vi "Multi U-Link DAQ Continuous value.vi"() -> ()   [LabVIEW 2017]
doc: "by Tanguy BOULARD"
uses:
  Type Def/Data.ctl
  <vilib>/Analysis/NI_AALBase.lvlib
panel:
  out "Energie IR file (500pts)":refnum<file>
  out "Puissance depolar file (500pts)":refnum<file>
  out "Energy UV file (500pts)":refnum<file>
  out "stop IR":bool
  out "stop Pd":bool
  out "stop UV":bool
  out "12sec IR":bool
  out "12sec Pd":bool
  out "12sec UV":bool
  out "Tableau IR":dbl[](array[numeric])
  out "Tableau UV":dbl[](array[numeric])
  out "Tableau Puissance depolar":dbl[](array[numeric])
  out "taille IR":dbl format="%.2f"
  out "taille Pd":dbl format="%.2f"
  out "taille UV":dbl format="%.2f"
  out "Energie IR mean":dbl caption="moyenne" format="%g"
  out "Energie IR variance":dbl caption="variance" format="%g"
  out "Energie IR max":dbl caption="max" format="%#_5g"
  out "Energie IR min":dbl caption="min"
  out "Puissance depolar mean":dbl caption="moyenne" format="%g"
  out "Puissance depolar variance":dbl caption="variance" format="%g"
  out "Puissance depolar max":dbl caption="max" format="%#_5g"
  out "Puissance depolar min":dbl caption="min" format="%#_5g"
  out "Energie UV mean":dbl caption="moyenne" format="%g"
  out "Energie UV variance":dbl caption="variance" format="%g"
  out "Energie UV max":dbl caption="max" format="%#_5g"
  out "Energie UV min":dbl caption="min" format="%#_5g"
  out "Energie UV rapport":dbl caption="rapport" format="%#_5g"
  out "Puissance depolar rapport":dbl caption="rapport" format="%#_5g"
  out "Energie IR rapport":dbl caption="rapport" format="%#_5g"
  out "Chaîne":string="Energie UV"
  out "Chaîne 2":string="Puissance depolar"
  out "Chaîne 3":string="Energie IR"
  out "sortie d'erreur":errorcluster caption="Sortie d'erreur"
  in  "stop":bool
  out "Energie IR value":dbl format="%#_4f"
  out "Energie IR graph":dbl(graph)
  out "Puissance depolar value":dbl format="%#_4f"
  out "Puissance depolar graph":dbl(graph)
  out "Energie IR table":dbl[](array[numeric])
  out "Energie IR table (1sec)":dbl[](array[numeric])
  out "Puissance depolar table":dbl[](array[numeric])
  out "Energie UV value":dbl format="%#_4f"
  out "Energie UV graph":dbl(graph)
  out "Energie UV table":dbl[](array[numeric])
  out "Energie UV table(1sec)":dbl[](array[numeric])
  out "Taux depolar value":dbl format="%#_4f"
  out "taux depolar graph":dbl(graph)
  out "Puissance depolar table (stats)":dbl[][](array[numeric])
  out "Energie IR table (stats)":dbl[][](array[numeric])
  out "Taux depolar indicator":u32(colorbox)=16777222
  out "Puissance depolar table (1sec)":dbl[](array[numeric])
  out "Energie UV table (stats)":dbl[][](array[numeric])
  out "timer 1sec":bool
  out "timer 12sec":bool
  in  "1sec":bool
  in  "12sec":bool
  out "index 1sec":i32
  out "index 12sec":i32
  out "Chaîne 4":string="Energie UV (mJ)"
  out "Chaîne 5":string="Energie IR (mJ)"
  out "Chaîne 6":string="Puissance depolar (W)"
  out "Chaîne 7":string="Taux depolar"
  out "Update":string="Initialization : matching U-Link ports, creating data file"
  in  "Start acquisition":bool
  in  "Commande onglets":T1(tab)
  out "Ressource VISA (Energie UV)":refnum<visa-resource-name>
  out "Wavelength (nm) (Energie UV)":u32=355
  out "Offset (Energie UV)":sgl
  out "Multiplier (Energie UV)":sgl=1.0
  out "Trigger Level (% of Scale) (Energie UV)":dbl=2.0 min=0.1 max=99.9 step=0.1 format="%_3f"
  out "Auto Scale (Energie UV)":bool=TRUE
  out "File name (Energie UV)":string="data.csv"
  out "Scale (Watt or Joule) (Energie UV)":i32(ring) items=["1 pico", "3 pico", "10 pico", "30 pico", "100 pico", "300 pico", "1 nano", "3 nano", "10 nano", "30 nano", "100 nano", "300 nano", "1 micro", "3 micro", "10 micro", "30 micro", "100 micro", "300 micro", "1 milli", "3 milli", "10 milli", "30 milli", "100 milli", "300 milli", "1", "3", "10", "30", "100", "300", "1 kilo", "3 kilo", "10 kilo", "30 kilo", "100 kilo", "300 kilo", "1 mega", "3 mega", "10 mega", "30 mega", "100 mega", "300 mega"]
  out "Ressource VISA (Puissance depolar)":refnum<visa-resource-name>
  out "Offset (Puissance depolar)":sgl
  out "Wavelength (nm) (Puissance depolar)":u32=1064
  out "Multiplier (Puissance depolar)":sgl=1.0
  out "Trigger Level (% of Scale) (Puissance depolar)":dbl=2.0 min=0.1 max=99.9 step=0.1 format="%_3f"
  out "Auto Scale (Puissance depolar)":bool=TRUE
  out "File name (Puissance depolar)":string="data.csv"
  out "Scale (Watt or Joule) (Puissance depolar)":u16(ring) items=["1 pico", "3 pico", "10 pico", "30 pico", "100 pico", "300 pico", "1 nano", "3 nano", "10 nano", "30 nano", "100 nano", "300 nano", "1 micro", "3 micro", "10 micro", "30 micro", "100 micro", "300 micro", "1 milli", "3 milli", "10 milli", "30 milli", "100 milli", "300 milli", "1", "3", "10", "30", "100", "300", "1 kilo", "3 kilo", "10 kilo", "30 kilo", "100 kilo", "300 kilo", "1 mega", "3 mega", "10 mega", "30 mega", "100 mega", "300 mega"]
  out "Ressource VISA (Energie IR)":refnum<visa-resource-name>
  out "Wavelength (nm) (Energie IR)":u32=1064
  out "Offset (Energie IR)":sgl
  out "Multiplier (Energie IR)":sgl=1.0
  out "Trigger Level (% of Scale) (Energie IR)":dbl=2.0 min=0.1 max=99.9 step=0.1 format="%_3f"
  out "File name (Energie IR)":string="data.csv"
  out "Scale (Watt or Joule) (Energie IR)":u16(ring) items=["1 pico", "3 pico", "10 pico", "30 pico", "100 pico", "300 pico", "1 nano", "3 nano", "10 nano", "30 nano", "100 nano", "300 nano", "1 micro", "3 micro", "10 micro", "30 micro", "100 micro", "300 micro", "1 milli", "3 milli", "10 milli", "30 milli", "100 milli", "300 milli", "1", "3", "10", "30", "100", "300", "1 kilo", "3 kilo", "10 kilo", "30 kilo", "100 kilo", "300 kilo", "1 mega", "3 mega", "10 mega", "30 mega", "100 mega", "300 mega"]
  out "Auto Scale (Energie IR)":bool
  out "error IO":errorcluster
  out "COM Port table":refnum<visa-resource-name>[](array[refnum])
  out "COM Port (Energie IR)":i64
  out "COM Port (Puissance depolar)":i64
  out "COM port (Energie UV)":i64
  out "User file contents Energie UV":dbl[](array[numeric])
  out "User file contents Energie IR":dbl[](array[numeric])
  out "User file contents Puissance depolar":dbl[](array[numeric])
  out "error?":bool caption="erreur ?"
  out "file path":path
  out "sortie d'erreur 3":errorcluster caption="sortie d'erreur"
  out "sortie d'erreur 2":errorcluster caption="sortie d'erreur"
  out "Energie UV file (1sec)":refnum<file>
  out "Energie UV file (stats)":refnum<file>
  out "Puissance depolar file (1sec)":refnum<file>
  out "Puissance depolar file (stats)":refnum<file>
  out "Energie IR file (1sec)":refnum<file>
  out "Energie IR file (stats)":refnum<file>
  in  "Bouton Accueil":bool
  out "chaîne de date/heure":string
  out "valeur de l'horloge en ms":u32
  out "Time":string
  out "stop?":bool=TRUE
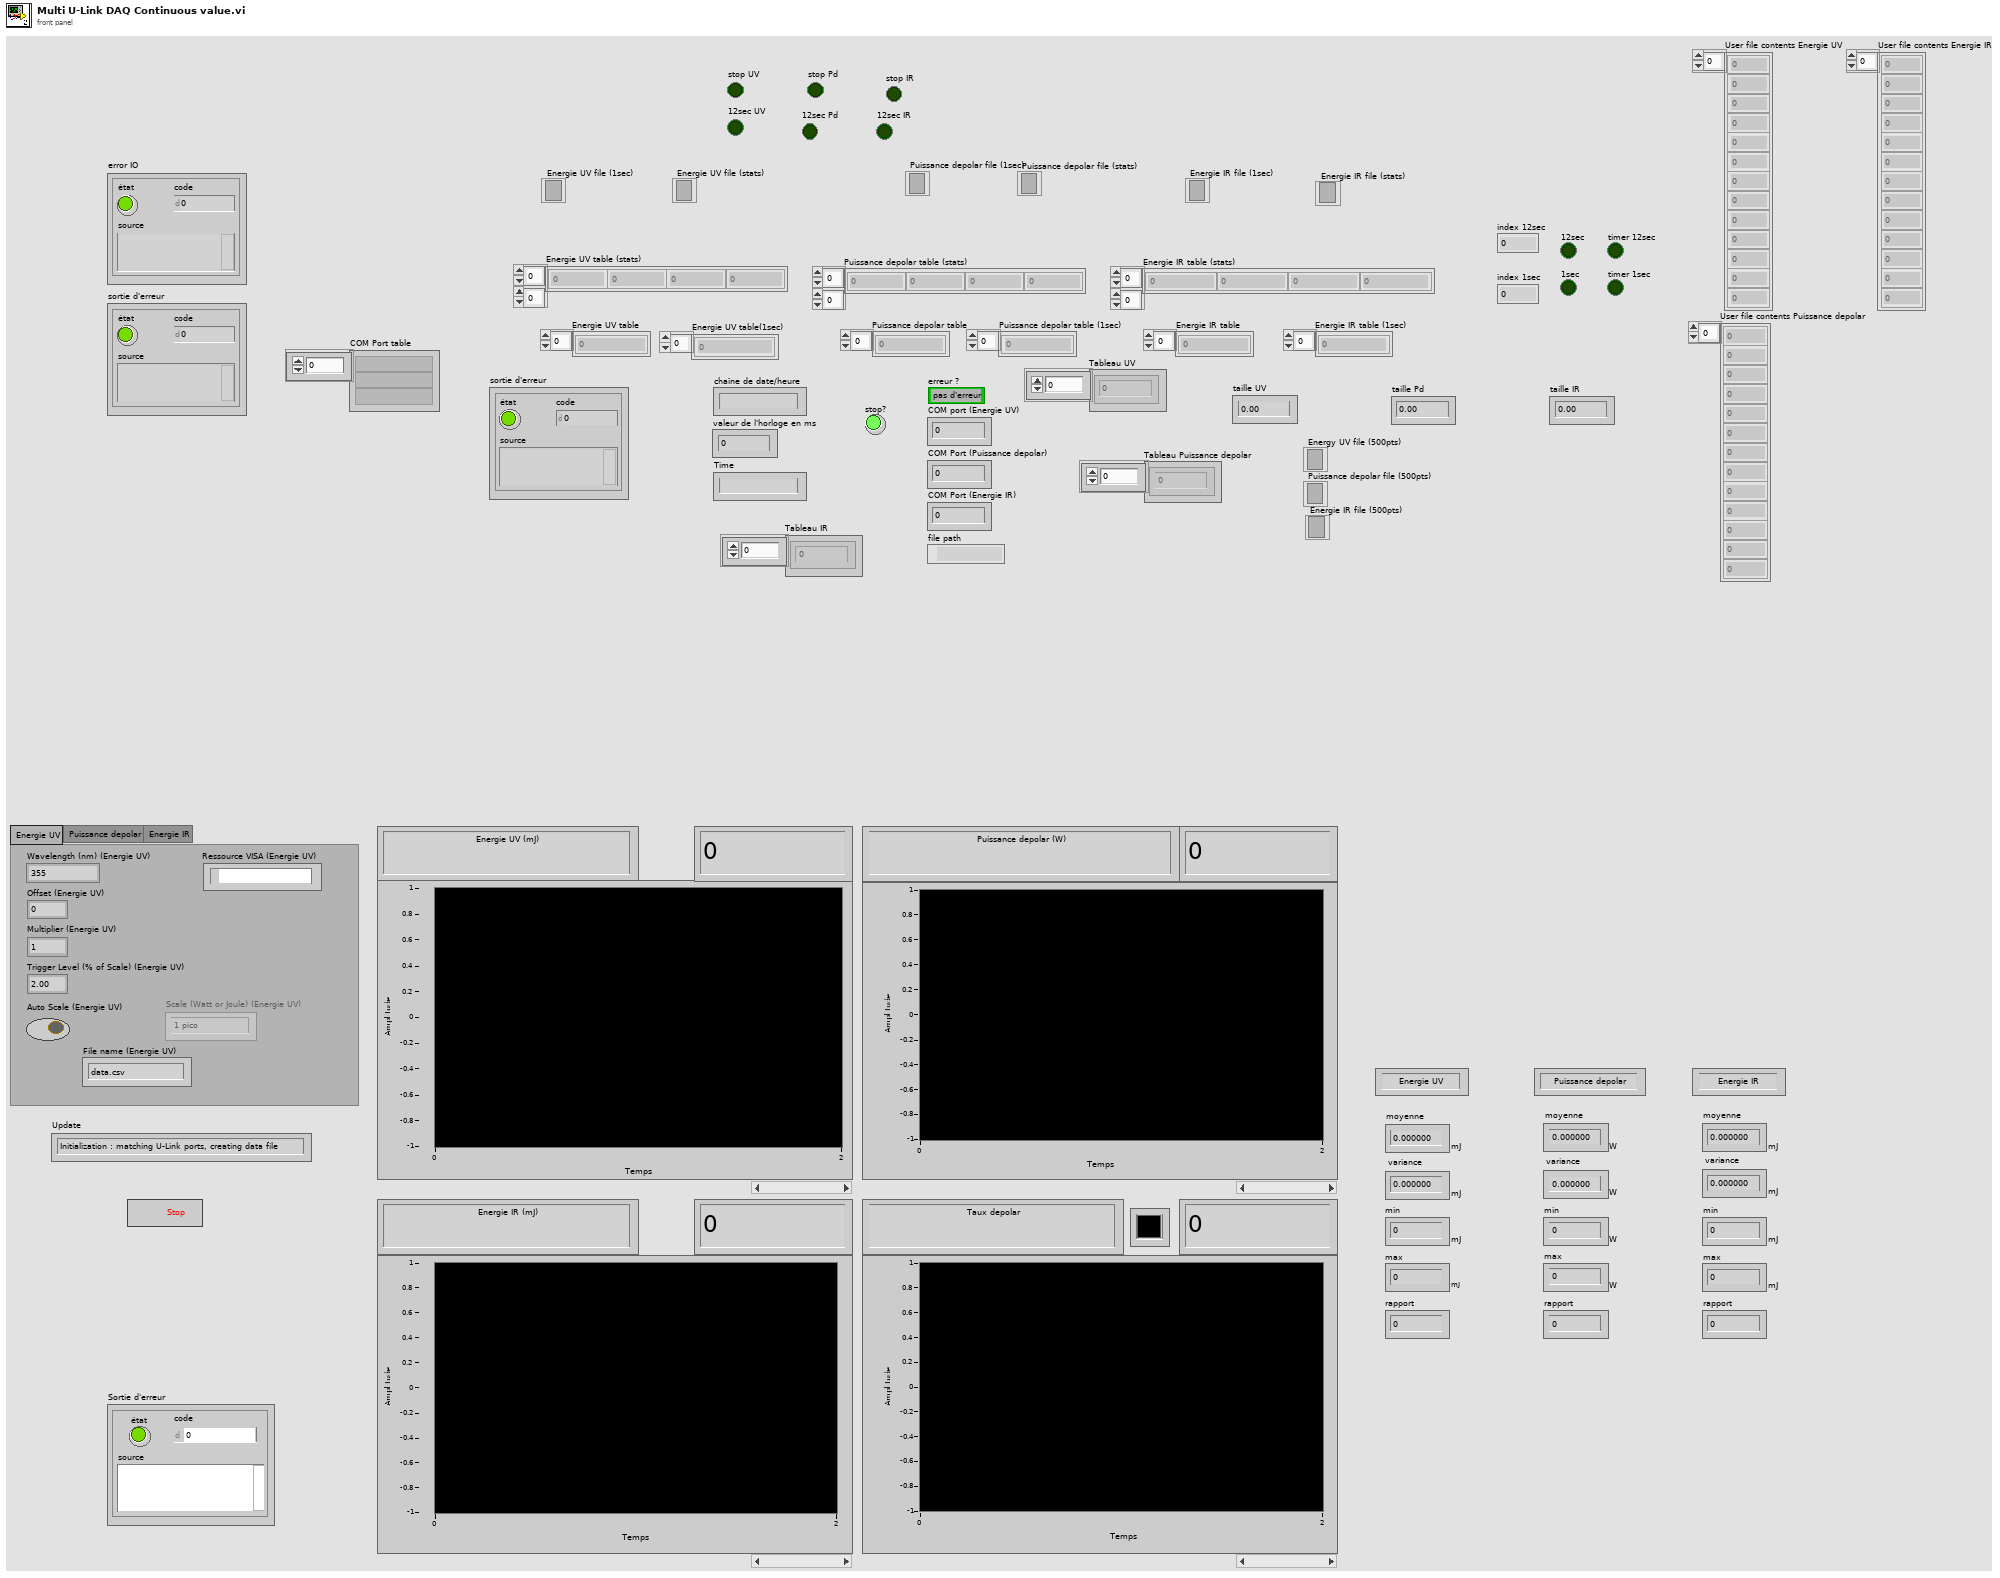
[diagram p1: front panel]
types:
  T1 = enum32{"Energie UV", "Puissance depolar", "Energie IR"}
  T2 = enum8{"Enabled", "Disabled", "Disabled and Grayed Out"}
  T3 = typedef "Data.ctl" = cluster{enum16{"Init", "Read", "Stop", "12sec"}, "Data":dbl}
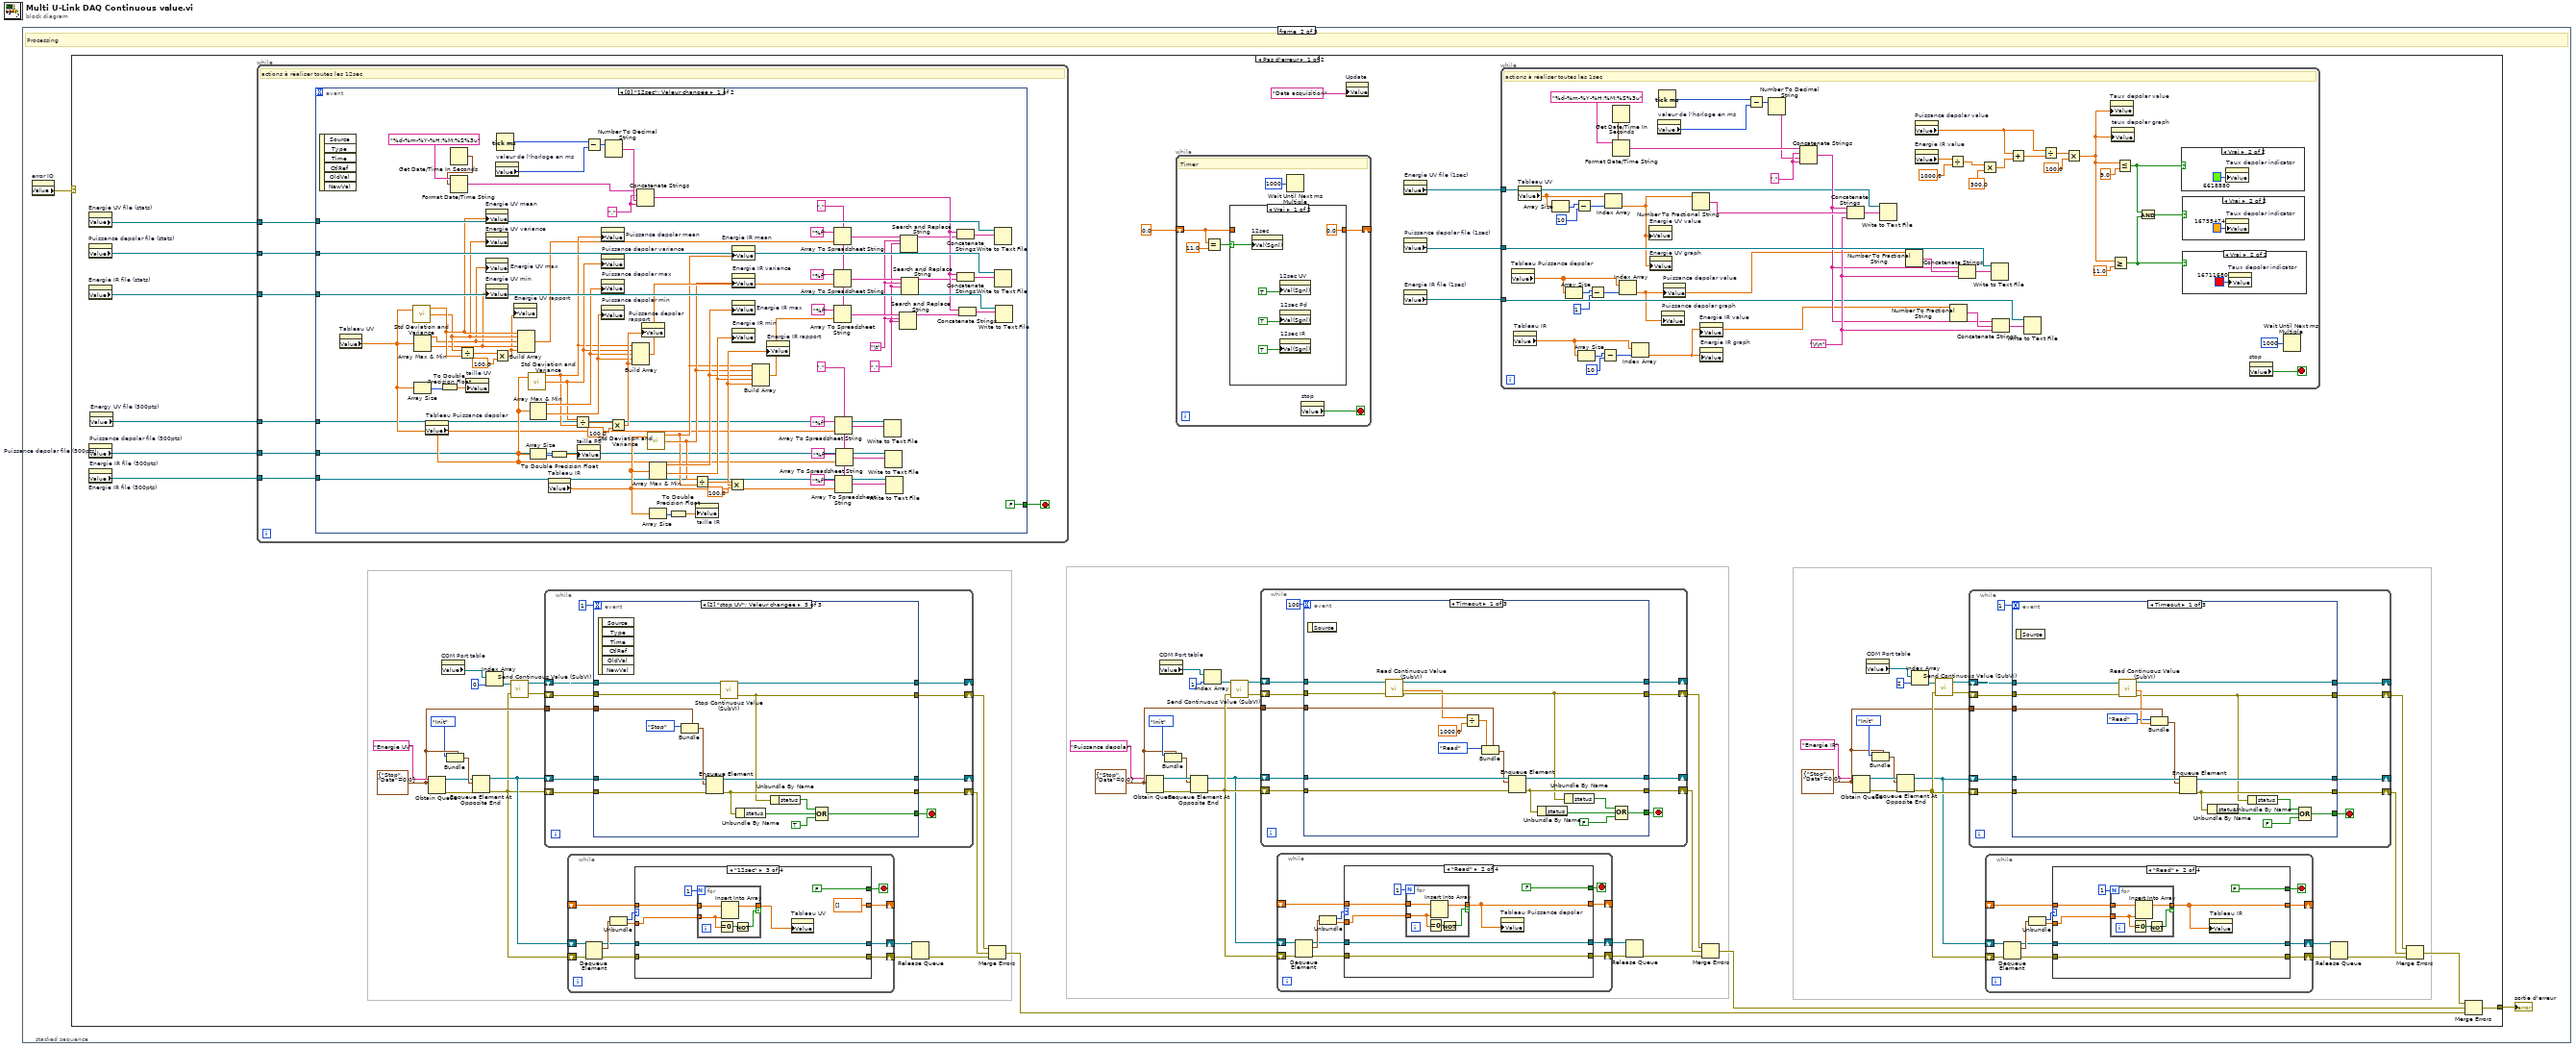
[diagram p0: block diagram]
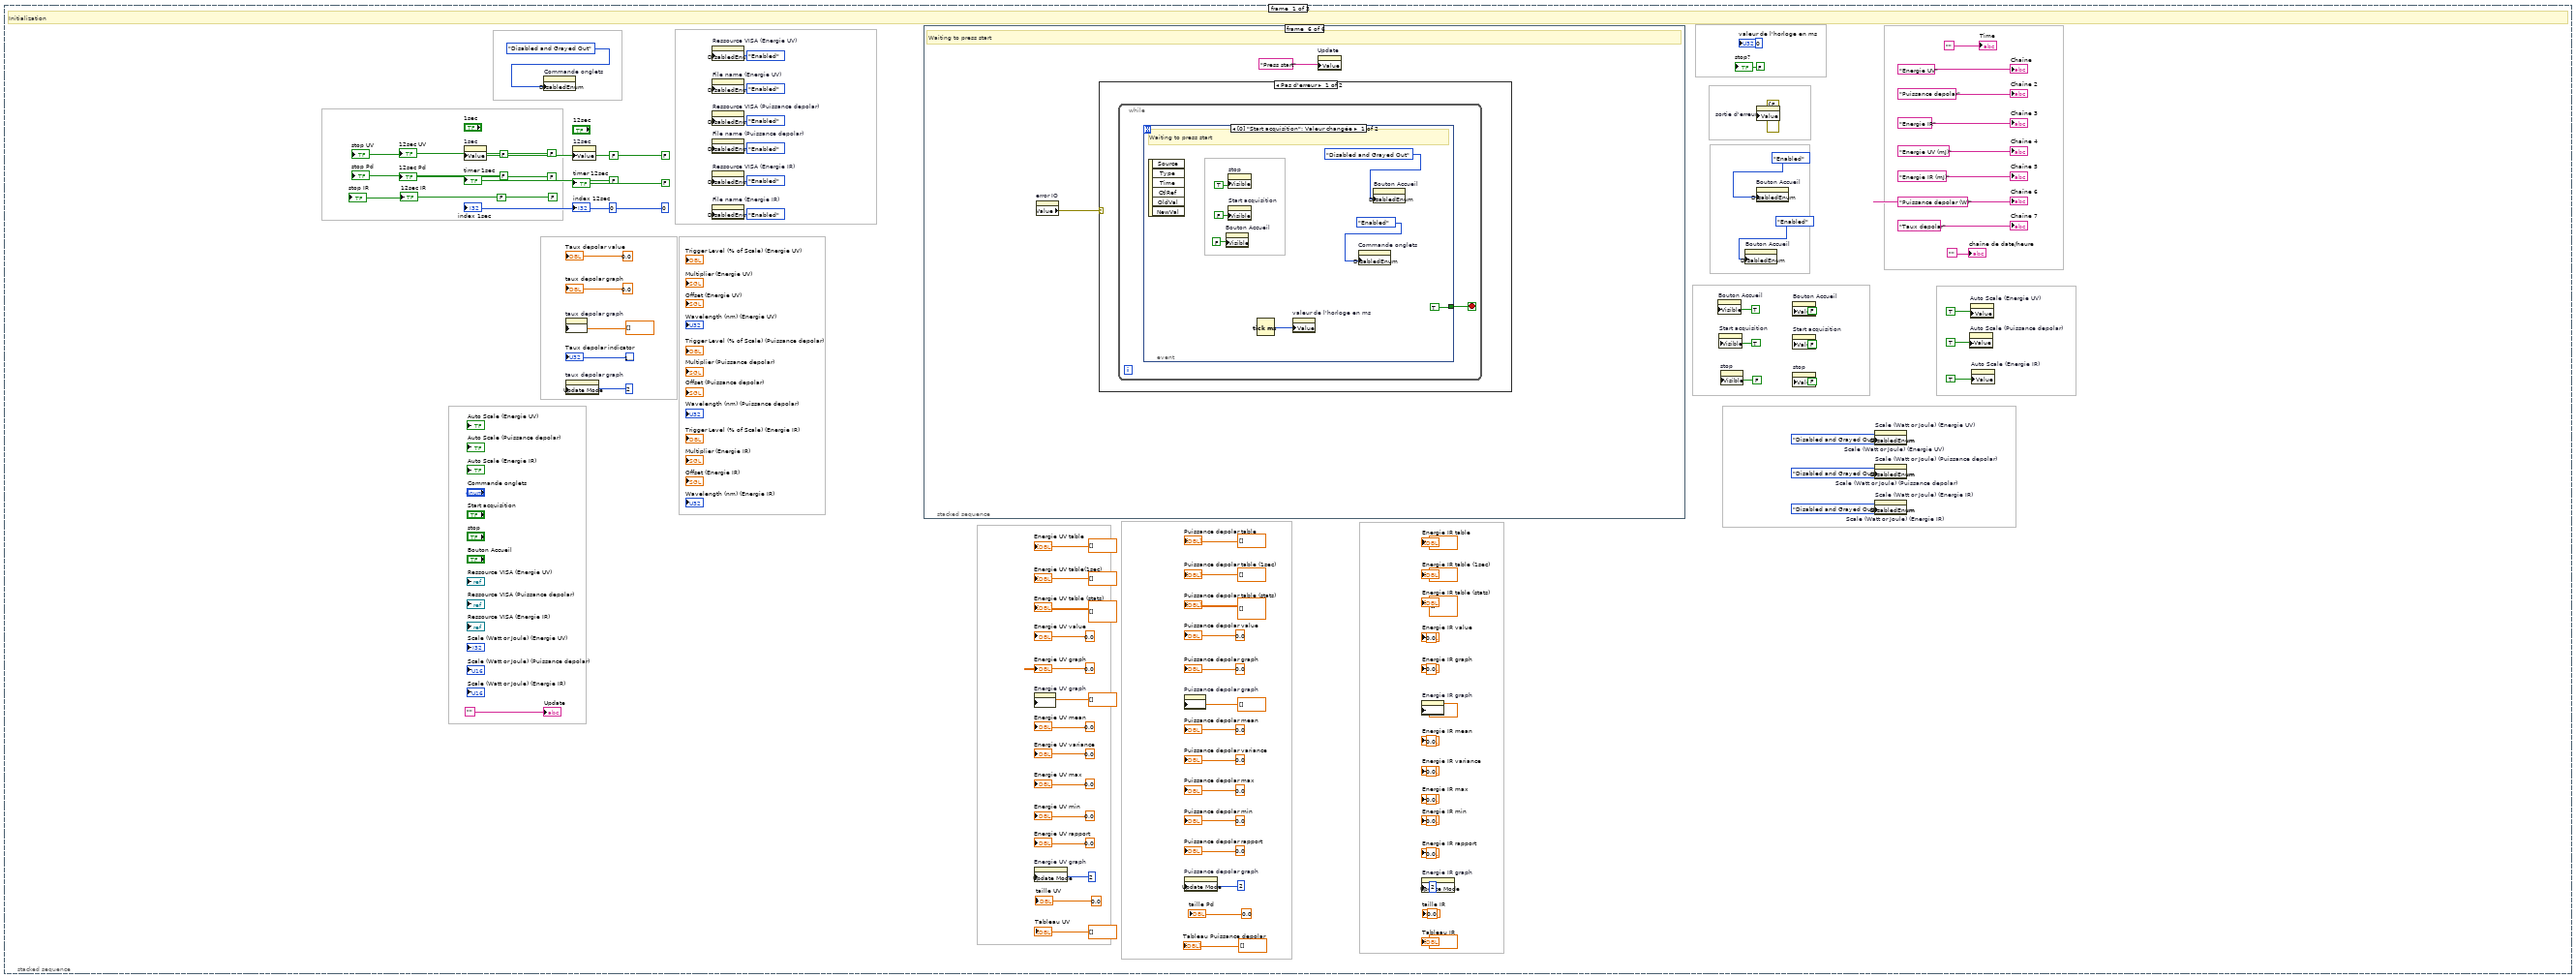
[diagram p2: hidden frame]
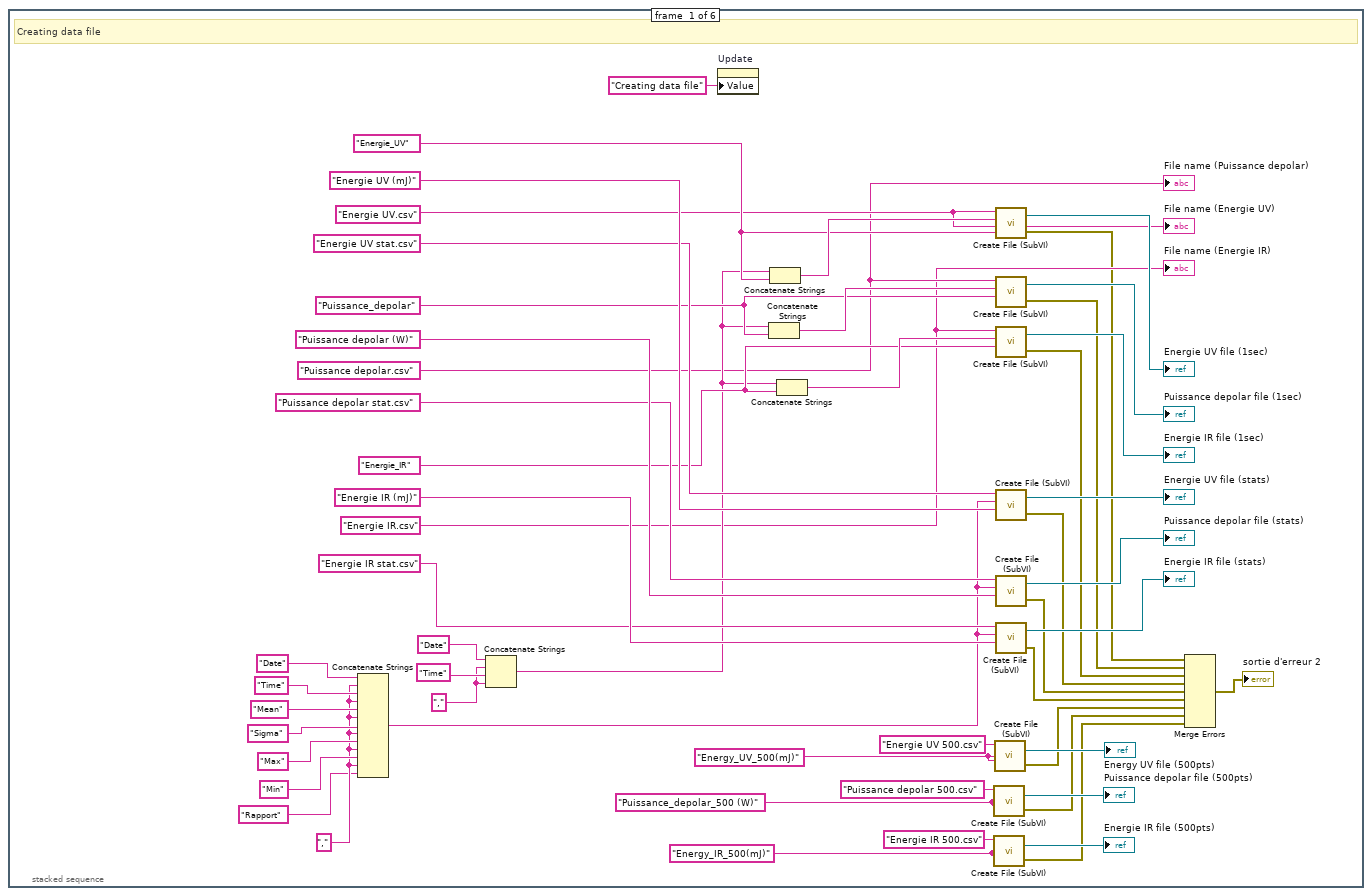
[diagram p3: hidden frame]
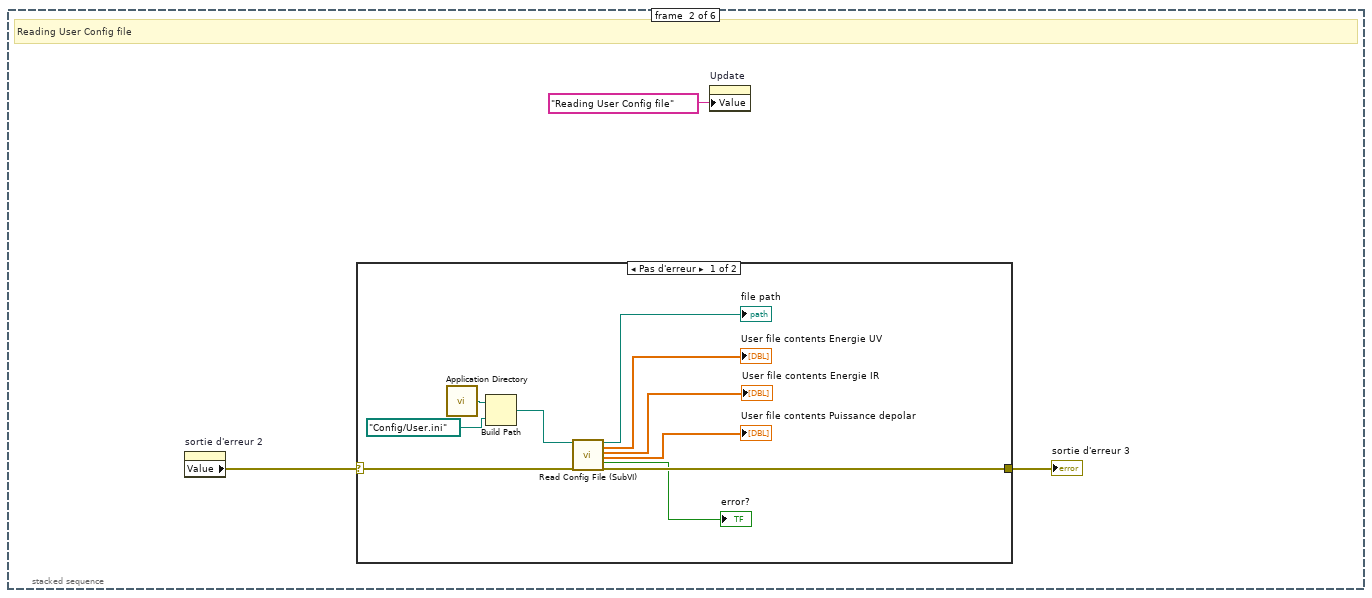
[diagram p4: hidden frame]
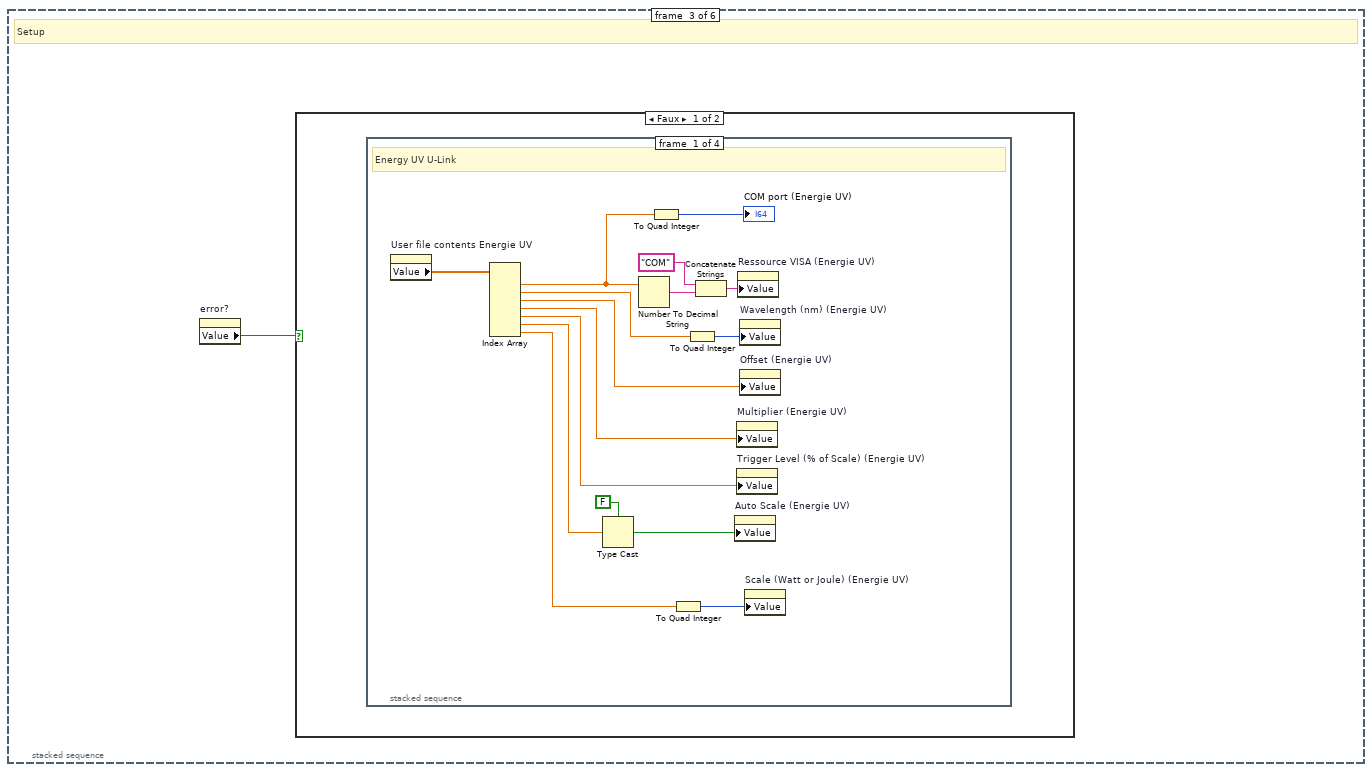
[diagram p6: hidden frame]
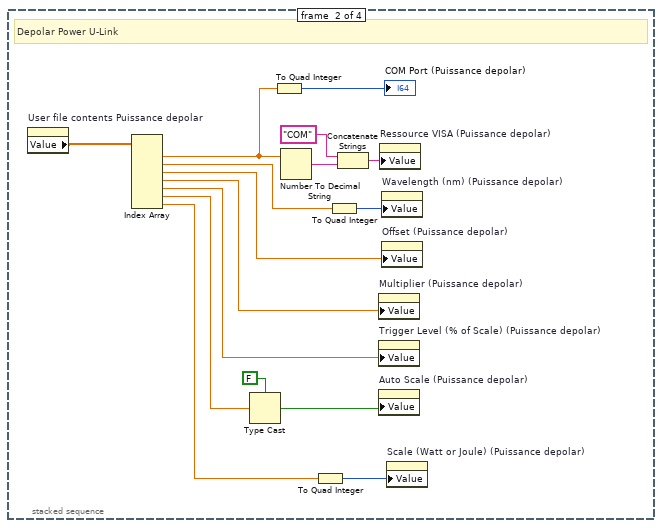
[diagram p7: hidden frame]
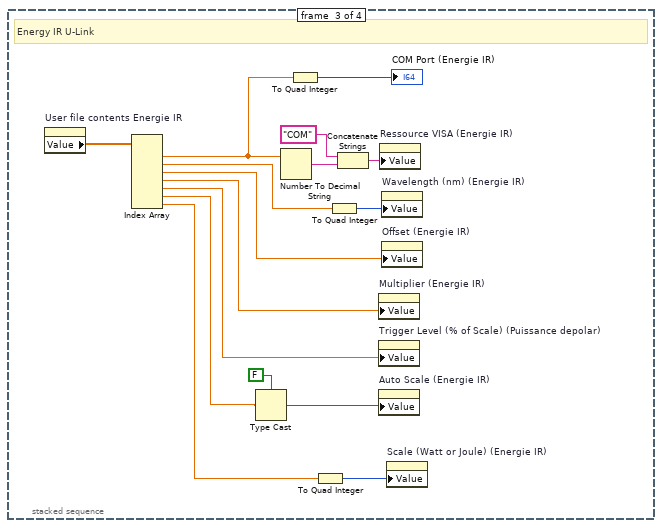
[diagram p8: hidden frame]
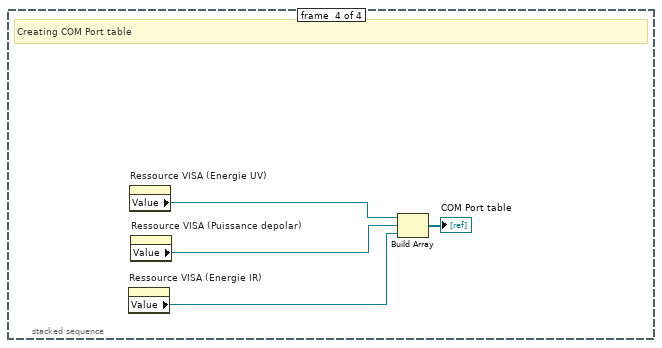
[diagram p9: hidden frame]
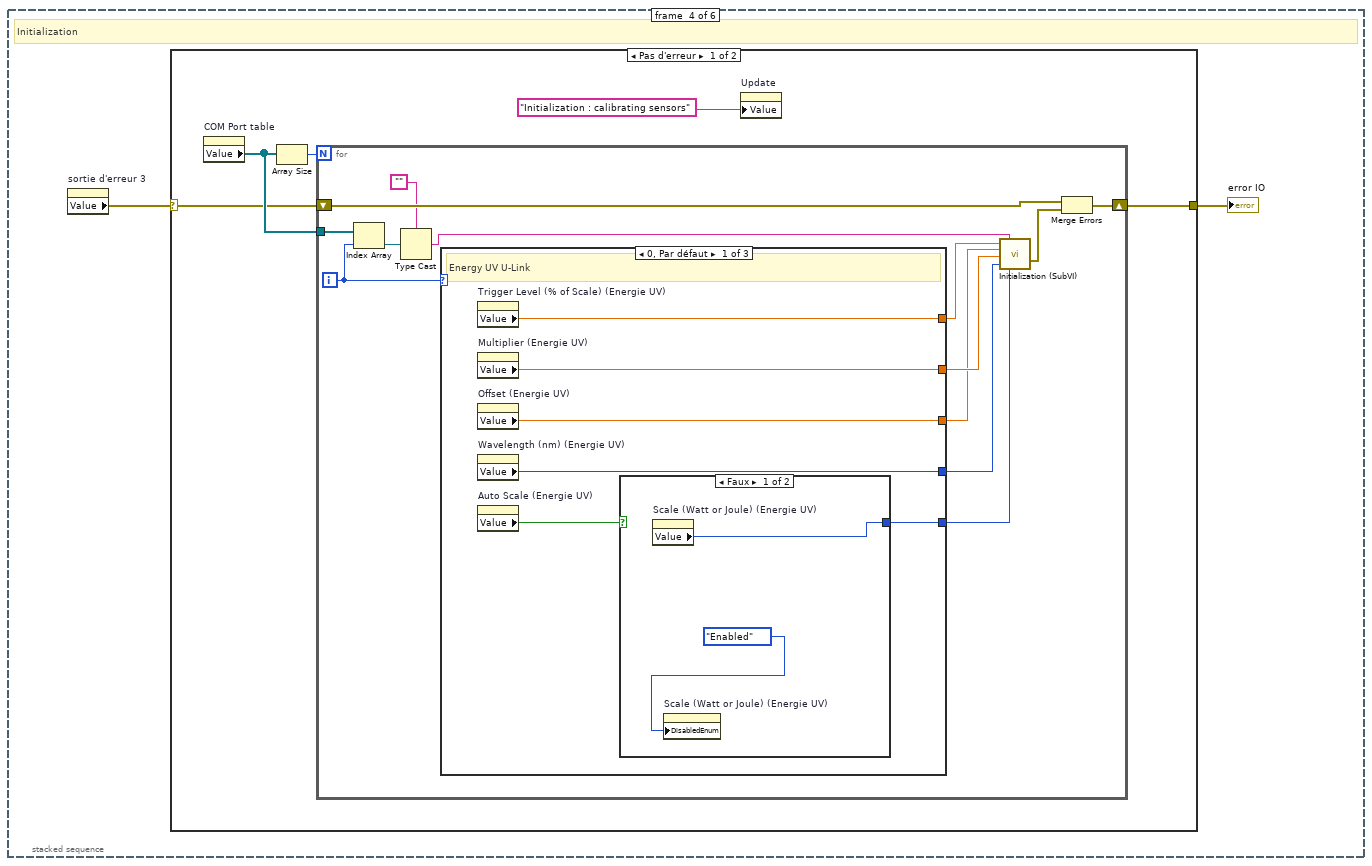
[diagram p11: hidden frame]
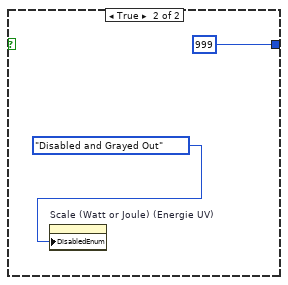
[diagram p12: hidden frame]
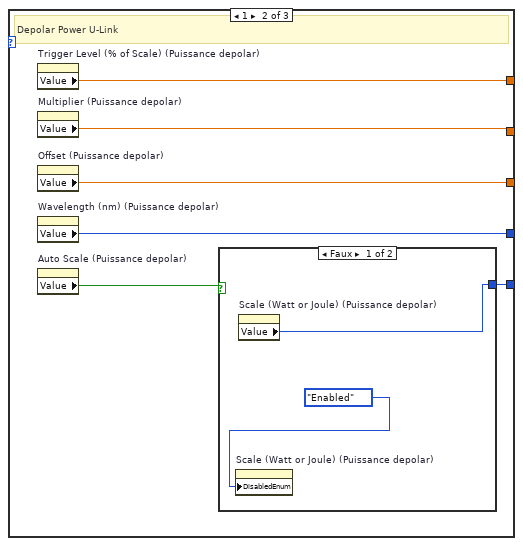
[diagram p13: hidden frame]
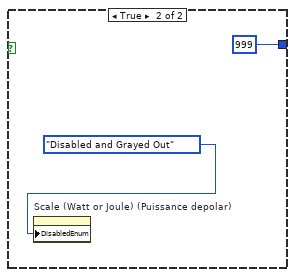
[diagram p14: hidden frame]
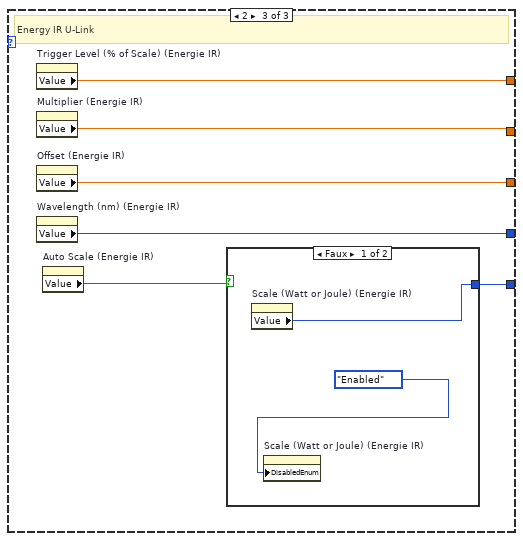
[diagram p15: hidden frame]
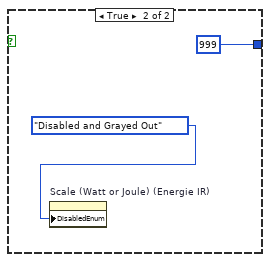
[diagram p16: hidden frame]
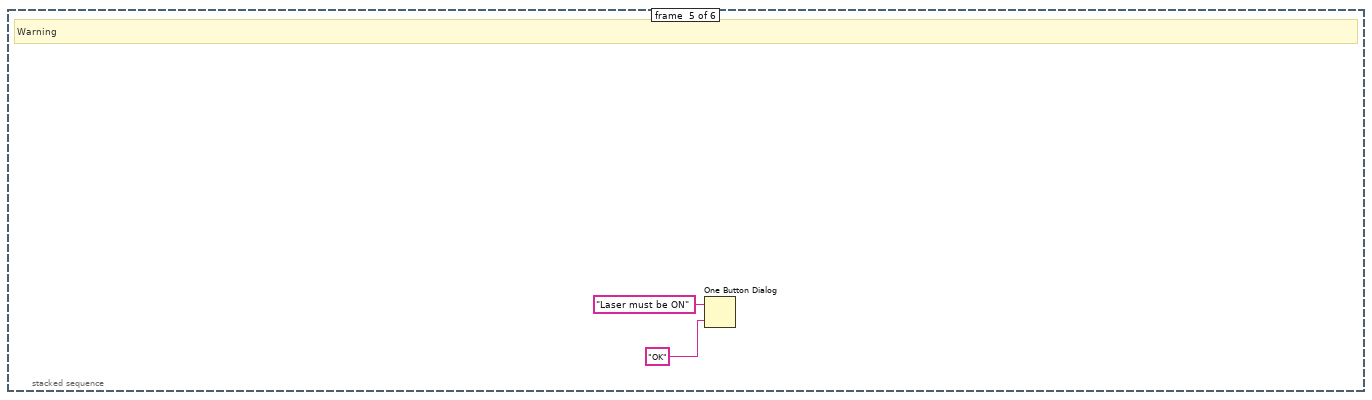
[diagram p18: hidden frame]
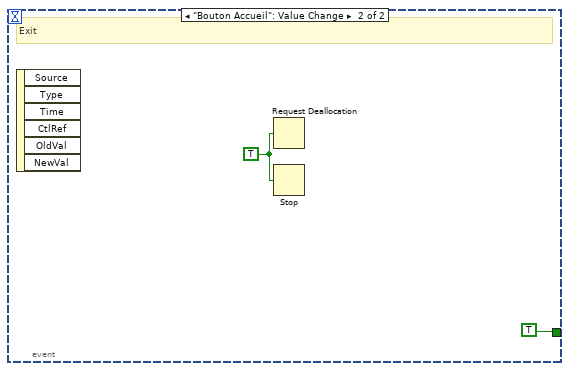
[diagram p19: hidden frame]
diagram:
  n1 = stacked-sequence {
    frame #0 {
      # "Initialization"
      n2 = property on="1sec" class="Bool (strict)"("Value"=FALSE ("1sec")) -> ()  [unwired: 2 in, 2 out]
      n3 = property on="Commande onglets" class="Onglet (strict)"("DisabledEnum"=T2."Disabled and Grayed Out" ("Désactivé")) -> ()  [unwired: 2 in, 2 out]
      n4 = property on="taux depolar graph" class="GraphDér (strict)"("History Data"=dbl[] [] ("Données d'historique")) -> ()  [unwired: 2 in, 2 out]
      n5 = property on="taux depolar graph" class="GraphDér (strict)"("Update Mode"=u8 2 ("Mode de rafraîchissement")) -> ()  [unwired: 2 in, 2 out]
      n6 = property on="12sec" class="Bool (strict)"("Value"=FALSE ("12sec")) -> ()  [unwired: 2 in, 2 out]
      n7 = property on="Ressource VISA (Energie UV)" class="NomVISA"("DisabledEnum"=T2."Enabled" ("Désactivé")) -> ()  [unwired: 2 in, 2 out]
      n8 = property on="File name (Energie UV)" class="Ch"("DisabledEnum"=T2."Enabled" ("Désactivé")) -> ()  [unwired: 2 in, 2 out]
      n9 = property on="Ressource VISA (Puissance depolar)" class="NomVISA"("DisabledEnum"=T2."Enabled" ("Désactivé")) -> ()  [unwired: 2 in, 2 out]
      n10 = property on="File name (Puissance depolar)" class="Ch"("DisabledEnum"=T2."Enabled" ("Désactivé")) -> ()  [unwired: 2 in, 2 out]
      n11 = property on="Ressource VISA (Energie IR)" class="NomVISA"("DisabledEnum"=T2."Enabled" ("Désactivé")) -> ()  [unwired: 2 in, 2 out]
      n12 = property on="File name (Energie IR)" class="Ch"("DisabledEnum"=T2."Enabled" ("Désactivé")) -> ()  [unwired: 2 in, 2 out]
      n13 = stacked-sequence {
        frame #0 {
          w104 = "Energy_IR_500(mJ)" ("data name")
          w105 = "Puissance_depolar_500 (W)" ("data name")
          w103 = "Energy_UV_500(mJ)" ("data name")
          w126 = ","
          w116 = ","
          w117 = "Energie IR.csv" ("file name 2")
          w121 = "Energie_IR" ("data name")
          w118 = "Puissance depolar.csv" ("file name 2")
          w123 = "Puissance_depolar" ("data name")
          w119 = "Energie UV.csv" ("file name")
          w128 = "Energie_UV" ("data name")
          # "Creating data file"
          n14 = Concatenate Strings("Date", w116, "Time", w116, "Mean", w116, "Sigma", w116, "Max", w116, "Min", w116, "Rapport" ("chaîne")) -> (w132:string)
          n15 = Concatenate Strings("Date", w126, "Time", w126) -> (w120:string)
          n16 = property on="Update" class="Ch"("Value"="Creating data file" ("Étiquette.Texte")) -> ()  [unwired: 2 in, 2 out]
          n17 = Concatenate Strings(w120, w123) -> (w124:string)
          n18 = Concatenate Strings(w120, w128) -> (w129:string)
          n19 = Concatenate Strings(w120, w121) -> (w122:string)
          n20 = call "Create File (SubVI).vi"("headers"=w105, "data name"=w105, "file name"="Puissance depolar 500.csv") -> ("error out"=w98:errorcluster, "Byte Stream File out"=→"Puissance depolar file (500pts)":refnum<file>)  [unwired: 1 in]
          n21 = call "Create File (SubVI).vi"("headers"=w104, "data name"=w104, "file name"="Energie IR 500.csv") -> ("error out"=w99:errorcluster, "Byte Stream File out"=→"Energie IR file (500pts)":refnum<file>)  [unwired: 1 in]
          n22 = call "Create File (SubVI).vi"("headers"=w103, "data name"=w103, "file name"="Energie UV 500.csv") -> ("error out"=w97:errorcluster, "Byte Stream File out"=→"Energy UV file (500pts)":refnum<file>)  [unwired: 1 in]
          n23 = call "Create File (SubVI).vi"("headers"=w128, "data name"=w129, "file name"=w119) -> ("error out"=w109:errorcluster, "Byte Stream File out"=→"Energie UV file (1sec)":refnum<file>)  [unwired: 1 in]
          n24 = call "Create File (SubVI).vi"("headers"=w123, "data name"=w124, "file name"=w118) -> ("error out"=w110:errorcluster, "Byte Stream File out"=→"Puissance depolar file (1sec)":refnum<file>)  [unwired: 1 in]
          n25 = call "Create File (SubVI).vi"("headers"=w121, "data name"=w122, "file name"=w117) -> ("error out"=w111:errorcluster, "Byte Stream File out"=→"Energie IR file (1sec)":refnum<file>)  [unwired: 1 in]
          n26 = call "Create File (SubVI).vi"("headers"="Energie UV (mJ)" ("data name"), "data name"=w132, "file name"="Energie UV stat.csv") -> ("error out"=w112:errorcluster, "Byte Stream File out"=→"Energie UV file (stats)":refnum<file>)  [unwired: 1 in]
          n27 = call "Create File (SubVI).vi"("headers"="Puissance depolar (W)" ("data name"), "data name"=w132, "file name"="Puissance depolar stat.csv" ("file name 2")) -> ("error out"=w113:errorcluster, "Byte Stream File out"=→"Puissance depolar file (stats)":refnum<file>)  [unwired: 1 in]
          n28 = call "Create File (SubVI).vi"("headers"="Energie IR (mJ)" ("data name"), "data name"=w132, "file name"="Energie IR stat.csv" ("file name 2")) -> ("error out"=w114:errorcluster, "Byte Stream File out"=→"Energie IR file (stats)":refnum<file>)  [unwired: 1 in]
          n29 = Merge Errors(w109, w110, w111, w112, w113, w114, w97, w98, w99) -> (→"sortie d'erreur 2":errorcluster)
          "File name (Energie UV)" <- w119
          "File name (Puissance depolar)" <- w118
          "File name (Energie IR)" <- w117
        }
        frame #1 {
          # "Reading User Config file"
          n30 = property on="sortie d'erreur 2" class="Clust (strict)"() -> ("Value"=w153:errorcluster)  [unwired: 2 in, 2 out]
          n31 = case shown="Pas d'erreur" w153 {
            selector: w153 -> [w162 w164]
            tunnel: [w163 w164] -> w152
            frame No Error {
              n32 = call <vilib>:"Application Directory.vi"() -> ("Application Directory"=w158:path)
              n33 = Build Path(base path=w158, name or relative path=path "Config/User.ini") -> (appended path=w156:path)
              n34 = call "Read Config File (SubVI).vi"("configuration file path"=w156, "entrée d'erreur (pas d'erreur)"=w162) -> ("file path"=→"file path":path, "User file contents Energie UV"=→"User file contents Energie UV":dbl[], "User file contents Energie IR"=→"User file contents Energie IR":dbl[], "User file contents Puissance depolar"=→"User file contents Puissance depolar":dbl[], "error?"=→"error?":bool, "sortie d'erreur"=w163:errorcluster)  [unwired: 12 in]
            }
            frame Error {
            }
          }
          "sortie d'erreur 3" <- w152
          n35 = property on="Update" class="Ch"("Value"="Reading User Config file" ("Étiquette.Texte")) -> ()  [unwired: 2 in, 2 out]
        }
        frame #2 {
          # "Setup"
          n36 = property on="error?" class="Bool (strict)"() -> ("Value"=w165:bool)  [unwired: 2 in, 2 out]
          n37 = case shown="Faux" w165 {
            frame False {
              n38 = stacked-sequence {
                frame #0 {
                  # "Energy UV U-Link"
                  n39 = property on="User file contents Energie UV" class="Tabl (strict)"() -> ("Value"=w166:dbl[])  [unwired: 2 in, 2 out]
                  n40 = Index Array(array=w166) -> (element #1=w178:dbl, element #2=w177:dbl, element #3=w175:dbl, element #4=w174:dbl, element #5=w169:dbl, element #6=w168:dbl, element #7=w167:dbl)  [unwired: 7 in]
                  n41 = Type Cast(type=FALSE, x=w168) -> (*(type *) &x=w171:bool)
                  n42 = Number To Decimal String(number=w178) -> (decimal integer string=w180:string)  [unwired: 1 in]
                  n43 = To Quad Integer(1:w178) -> (0:→"COM port (Energie UV)":i64)
                  n44 = To Quad Integer(1:w167) -> (0:w173:i64)
                  n45 = To Quad Integer(1:w177) -> (0:w176:i64)
                  n46 = Concatenate Strings("COM" ("string"), w180) -> (w179:string)
                  n47 = property on="Auto Scale (Energie UV)" class="Bool (strict)"("Value"=w171) -> ()  [unwired: 2 in, 2 out]
                  n48 = property on="Multiplier (Energie UV)" class="NumNb (strict)"("Value"=w174) -> ()  [unwired: 2 in, 2 out]
                  n49 = property on="Trigger Level (% of Scale) (Energie UV)" class="NumNb (strict)"("Value"=w169) -> ()  [unwired: 2 in, 2 out]
                  n50 = property on="Ressource VISA (Energie UV)" class="NomVISA"("Value"=w179) -> ()  [unwired: 2 in, 2 out]
                  n51 = property on="Wavelength (nm) (Energie UV)" class="NumNb (strict)"("Value"=w176) -> ()  [unwired: 2 in, 2 out]
                  n52 = property on="Offset (Energie UV)" class="NumNb (strict)"("Value"=w175) -> ()  [unwired: 2 in, 2 out]
                  n53 = property on="Scale (Watt or Joule) (Energie UV)" class="MDér (strict)"("Value"=w173) -> ()  [unwired: 2 in, 2 out]
                }
                frame #1 {
                  # "Depolar Power U-Link"
                  n54 = property on="User file contents Puissance depolar" class="Tabl (strict)"() -> ("Value"=w188:dbl[])  [unwired: 2 in, 2 out]
                  n55 = Index Array(array=w188) -> (element #1=w194:dbl, element #2=w193:dbl, element #3=w191:dbl, element #4=w190:dbl, element #5=w184:dbl, element #6=w183:dbl, element #7=w182:dbl)  [unwired: 7 in]
                  n56 = Type Cast(type=FALSE, x=w183) -> (*(type *) &x=w185:bool)
                  n57 = To Quad Integer(1:w194) -> (0:→"COM Port (Puissance depolar)":i64)
                  n58 = Number To Decimal String(number=w194) -> (decimal integer string=w196:string)  [unwired: 1 in]
                  n59 = To Quad Integer(1:w182) -> (0:w189:i64)
                  n60 = To Quad Integer(1:w193) -> (0:w192:i64)
                  n61 = Concatenate Strings("COM" ("string"), w196) -> (w195:string)
                  n62 = property on="Multiplier (Puissance depolar)" class="NumNb (strict)"("Value"=w190) -> ()  [unwired: 2 in, 2 out]
                  n63 = property on="Trigger Level (% of Scale) (Puissance depolar)" class="NumNb (strict)"("Value"=w184) -> ()  [unwired: 2 in, 2 out]
                  n64 = property on="Auto Scale (Puissance depolar)" class="Bool (strict)"("Value"=w185) -> ()  [unwired: 2 in, 2 out]
                  n65 = property on="Ressource VISA (Puissance depolar)" class="NomVISA"("Value"=w195) -> ()  [unwired: 2 in, 2 out]
                  n66 = property on="Wavelength (nm) (Puissance depolar)" class="NumNb (strict)"("Value"=w192) -> ()  [unwired: 2 in, 2 out]
                  n67 = property on="Offset (Puissance depolar)" class="NumNb (strict)"("Value"=w191) -> ()  [unwired: 2 in, 2 out]
                  n68 = property on="Scale (Watt or Joule) (Puissance depolar)" class="MDér (strict)"("Value"=w189) -> ()  [unwired: 2 in, 2 out]
                }
                frame #2 {
                  # "Energy IR U-Link"
                  n69 = property on="User file contents Energie IR" class="Tabl (strict)"() -> ("Value"=w204:dbl[])  [unwired: 2 in, 2 out]
                  n70 = Index Array(array=w204) -> (element #1=w210:dbl, element #2=w209:dbl, element #3=w207:dbl, element #4=w206:dbl, element #5=w200:dbl, element #6=w199:dbl, element #7=w198:dbl)  [unwired: 7 in]
                  n71 = Type Cast(type=FALSE, x=w199) -> (*(type *) &x=w202:bool)
                  n72 = Number To Decimal String(number=w210) -> (decimal integer string=w212:string)  [unwired: 1 in]
                  n73 = To Quad Integer(1:w210) -> (0:→"COM Port (Energie IR)":i64)
                  n74 = To Quad Integer(1:w198) -> (0:w205:i64)
                  n75 = To Quad Integer(1:w209) -> (0:w208:i64)
                  n76 = Concatenate Strings("COM" ("string"), w212) -> (w211:string)
                  n77 = property on="Multiplier (Energie IR)" class="NumNb (strict)"("Value"=w206) -> ()  [unwired: 2 in, 2 out]
                  n78 = property on="Trigger Level (% of Scale) (Puissance depolar)" class="NumNb (strict)"("Value"=w200) -> ()  [unwired: 2 in, 2 out]
                  n79 = property on="Auto Scale (Energie IR)" class="Bool (strict)"("Value"=w202) -> ()  [unwired: 2 in, 2 out]
                  n80 = property on="Ressource VISA (Energie IR)" class="NomVISA"("Value"=w211) -> ()  [unwired: 2 in, 2 out]
                  n81 = property on="Wavelength (nm) (Energie IR)" class="NumNb (strict)"("Value"=w208) -> ()  [unwired: 2 in, 2 out]
                  n82 = property on="Offset (Energie IR)" class="NumNb (strict)"("Value"=w207) -> ()  [unwired: 2 in, 2 out]
                  n83 = property on="Scale (Watt or Joule) (Energie IR)" class="MDér (strict)"("Value"=w205) -> ()  [unwired: 2 in, 2 out]
                }
                frame #3 {
                  # "Creating COM Port table"
                  n84 = property on="Ressource VISA (Energie IR)" class="NomVISA"() -> ("Value"=w217:refnum<visa-resource-name>)  [unwired: 2 in, 2 out]
                  n85 = property on="Ressource VISA (Energie UV)" class="NomVISA"() -> ("Value"=w215:refnum<visa-resource-name>)  [unwired: 2 in, 2 out]
                  n86 = property on="Ressource VISA (Puissance depolar)" class="NomVISA"() -> ("Value"=w216:refnum<visa-resource-name>)  [unwired: 2 in, 2 out]
                  n87 = Build Array(w215, w216, w217) -> (→"COM Port table":refnum<visa-resource-name>[])
                }
              }
            }
            frame True {
            }
          }
        }
        frame #3 {
          # "Initialization"
          n88 = property on="sortie d'erreur 3" class="Clust (strict)"() -> ("Value"=w218:errorcluster)  [unwired: 2 in, 2 out]
          n89 = case shown="Pas d'erreur" w218 {
            selector: w218 -> [w220 w268]
            tunnel: [w223 w268] -> w219
            frame No Error {
              n90 = property on="COM Port table" class="Tabl (strict)"() -> ("Value"=w221:refnum<visa-resource-name>[])  [unwired: 2 in, 2 out]
              n91 = Array Size(array=w221) -> (size(s)=w222:i32)
              n92 = for {
                N: w222 -> [_]
                shift-right: [w231] -> w223
                shift-left: w220 -> [w230]
                tunnel: w221 -> [w225]
                i -> [w226]
                n93 = Index Array(array=w225, index=w226) -> (element=w228:refnum<visa-resource-name>)
                n94 = Type Cast(type="", x=w228) -> (*(type *) &x=w229:string)
                n95 = case shown="0, Par défaut" w226 {
                  tunnel: [w243 w250 w260] -> w237
                  tunnel: [w240 w251 w261] -> w235
                  tunnel: [w242 w252 w262] -> w236
                  tunnel: [w241 w253 w263] -> w234
                  tunnel: [w239 w249 w259] -> w233
                  frame 0, Default {
                    # "Energy UV U-Link"
                    n96 = property on="Trigger Level (% of Scale) (Energie UV)" class="NumNb (strict)"() -> ("Value"=w241:dbl)  [unwired: 2 in, 2 out]
                    n97 = property on="Multiplier (Energie UV)" class="NumNb (strict)"() -> ("Value"=w242:sgl)  [unwired: 2 in, 2 out]
                    n98 = property on="Offset (Energie UV)" class="NumNb (strict)"() -> ("Value"=w240:sgl)  [unwired: 2 in, 2 out]
                    n99 = property on="Wavelength (nm) (Energie UV)" class="NumNb (strict)"() -> ("Value"=w243:u32)  [unwired: 2 in, 2 out]
                    n100 = property on="Auto Scale (Energie UV)" class="Bool (strict)"() -> ("Value"=w238:bool)  [unwired: 2 in, 2 out]
                    n101 = case shown="Faux" w238 {
                      tunnel: [w245 u32 999 ("Value")] -> w239
                      frame False {
                        n102 = property on="Scale (Watt or Joule) (Energie UV)" class="MDér (strict)"() -> ("Value"=w245:i32)  [unwired: 2 in, 2 out]
                        n103 = property on="Scale (Watt or Joule) (Energie UV)" class="MDér (strict)"("DisabledEnum"=T2."Enabled" ("Désactivé")) -> ()  [unwired: 2 in, 2 out]
                      }
                      frame True {
                        n104 = property on="Scale (Watt or Joule) (Energie UV)" class="MDér (strict)"("DisabledEnum"=T2."Disabled and Grayed Out" ("Désactivé")) -> ()  [unwired: 2 in, 2 out]
                      }
                    }
                  }
                  frame 1 {
                    # "Depolar Power U-Link"
                    n105 = property on="Trigger Level (% of Scale) (Puissance depolar)" class="NumNb (strict)"() -> ("Value"=w253:dbl)  [unwired: 2 in, 2 out]
                    n106 = property on="Multiplier (Puissance depolar)" class="NumNb (strict)"() -> ("Value"=w252:sgl)  [unwired: 2 in, 2 out]
                    n107 = property on="Offset (Puissance depolar)" class="NumNb (strict)"() -> ("Value"=w251:sgl)  [unwired: 2 in, 2 out]
                    n108 = property on="Wavelength (nm) (Puissance depolar)" class="NumNb (strict)"() -> ("Value"=w250:u32)  [unwired: 2 in, 2 out]
                    n109 = property on="Auto Scale (Puissance depolar)" class="Bool (strict)"() -> ("Value"=w248:bool)  [unwired: 2 in, 2 out]
                    n110 = case shown="Faux" w248 {
                      tunnel: [w255 u32 999 ("Value")] -> w249
                      frame False {
                        n111 = property on="Scale (Watt or Joule) (Puissance depolar)" class="MDér (strict)"("DisabledEnum"=T2."Enabled" ("Désactivé")) -> ()  [unwired: 2 in, 2 out]
                        n112 = property on="Scale (Watt or Joule) (Puissance depolar)" class="MDér (strict)"() -> ("Value"=w255:u16)  [unwired: 2 in, 2 out]
                      }
                      frame True {
                        n113 = property on="Scale (Watt or Joule) (Puissance depolar)" class="MDér (strict)"("DisabledEnum"=T2."Disabled and Grayed Out" ("Désactivé")) -> ()  [unwired: 2 in, 2 out]
                      }
                    }
                  }
                  frame 2 {
                    # "Energy IR U-Link"
                    n114 = property on="Trigger Level (% of Scale) (Energie IR)" class="NumNb (strict)"() -> ("Value"=w263:dbl)  [unwired: 2 in, 2 out]
                    n115 = property on="Multiplier (Energie IR)" class="NumNb (strict)"() -> ("Value"=w262:sgl)  [unwired: 2 in, 2 out]
                    n116 = property on="Offset (Energie IR)" class="NumNb (strict)"() -> ("Value"=w261:sgl)  [unwired: 2 in, 2 out]
                    n117 = property on="Wavelength (nm) (Energie IR)" class="NumNb (strict)"() -> ("Value"=w260:u32)  [unwired: 2 in, 2 out]
                    n118 = property on="Auto Scale (Energie IR)" class="Bool (strict)"() -> ("Value"=w258:bool)  [unwired: 2 in, 2 out]
                    n119 = case shown="Faux" w258 {
                      tunnel: [w265 u32 999 ("Value")] -> w259
                      frame False {
                        n120 = property on="Scale (Watt or Joule) (Energie IR)" class="MDér (strict)"() -> ("Value"=w265:u16)  [unwired: 2 in, 2 out]
                        n121 = property on="Scale (Watt or Joule) (Energie IR)" class="MDér (strict)"("DisabledEnum"=T2."Enabled" ("Désactivé")) -> ()  [unwired: 2 in, 2 out]
                      }
                      frame True {
                        n122 = property on="Scale (Watt or Joule) (Energie IR)" class="MDér (strict)"("DisabledEnum"=T2."Disabled and Grayed Out" ("Désactivé")) -> ()  [unwired: 2 in, 2 out]
                      }
                    }
                  }
                }
                n123 = call "Initialization (SubVI).vi"("Trigger Level (% of Scale)"=w234, "VISA Refnum in"=w229, "Offset"=w235, "Multiplier"=w236, "Wavelength (nm)"=w237, "Scale"=w233) -> ("error out"=w232:errorcluster)  [unwired: 8 in, 1 out]
                n124 = Merge Errors(w230, w232) -> (w231:errorcluster)
              }
              n125 = property on="Update" class="Ch"("Value"="Initialization : calibrating sensors" ("Étiquette.Texte")) -> ()  [unwired: 2 in, 2 out]
            }
            frame Error {
            }
          }
          "error IO" <- w219
        }
        frame #4 {
          # "Warning"
          n126 = One Button Dialog(message="Laser must be ON", button name ("OK")="OK" ("nom du bouton (\"OK\")")) -> ()  [unwired: 1 out]
        }
        frame #5 {
          # "Waiting to press start"
          n127 = property on="error IO" class="Clust (strict)"() -> ("Value"=w272:errorcluster)  [unwired: 2 in, 2 out]
          n128 = case shown="Pas d'erreur" w272 {
            frame No Error {
              n129 = while {
                stop <- w273 stop-if-true
                n130 = event "Structure Événement" shown="[0] \"Start acquisition\": Valeur changée" {
                  selector: _ -> [_ _]
                  dyn-events: _ -> [_ _]
                  timeout: _ -> [_ _]
                  tunnel: [TRUE TRUE] -> w273
                  event "Start acquisition": Value Change {
                    # "Waiting to press start"
                    n131 = event-data() -> ()  [unwired: 1 in, 6 out]
                    n132 = property on="Bouton Accueil" class="Bool (strict)"("Visible"=FALSE) -> ()  [unwired: 2 in, 2 out]
                    n133 = property on="stop" class="Bool (strict)"("Visible"=TRUE) -> ()  [unwired: 2 in, 2 out]
                    n134 = property on="Start acquisition" class="Bool (strict)"("Visible"=FALSE) -> ()  [unwired: 2 in, 2 out]
                    n135 = Tick Count (ms)() -> (millisecond timer value=w274:u32)
                    n136 = property on="valeur de l'horloge en ms" class="NumNb (strict)"("Value"=w274) -> ()  [unwired: 2 in, 2 out]
                    n137 = property on="Commande onglets" class="Onglet (strict)"("DisabledEnum"=T2."Enabled" ("Désactivé")) -> ()  [unwired: 2 in, 2 out]
                    n138 = property on="Bouton Accueil" class="Bool (strict)"("DisabledEnum"=T2."Disabled and Grayed Out" ("Désactivé")) -> ()  [unwired: 2 in, 2 out]
                  }
                  event "Bouton Accueil": Value Change {
                    w282 = TRUE ("flag")
                    # "Exit"
                    n139 = event-data() -> ()  [unwired: 1 in, 6 out]
                    n140 = Request Deallocation(w282) -> ()
                    n141 = Stop(stop? (T)=w282) -> ()
                  }
                }
              }
            }
            frame Error {
            }
          }
          n142 = property on="Update" class="Ch"("Value"="Press start" ("Étiquette.Texte")) -> ()  [unwired: 2 in, 2 out]
        }
      }
      n143 = property on="Energie UV graph" class="GraphDér (strict)"("History Data"=dbl[] [] ("Données d'historique")) -> ()  [unwired: 2 in, 2 out]
      n144 = property on="Energie UV graph" class="GraphDér (strict)"("Update Mode"=u8 2 ("Mode de rafraîchissement")) -> ()  [unwired: 2 in, 2 out]
      n145 = property on="Puissance depolar graph" class="GraphDér (strict)"("History Data"=dbl[] [] ("Données d'historique")) -> ()  [unwired: 2 in, 2 out]
      n146 = property on="Puissance depolar graph" class="GraphDér (strict)"("Update Mode"=u8 2 ("Mode de rafraîchissement")) -> ()  [unwired: 2 in, 2 out]
      n147 = property on="Energie IR graph" class="GraphDér (strict)"("History Data"=dbl[] [] ("Données d'historique")) -> ()  [unwired: 2 in, 2 out]
      n148 = property on="Energie IR graph" class="GraphDér (strict)"("Update Mode"=u8 2 ("Mode de rafraîchissement")) -> ()  [unwired: 2 in, 2 out]
      n149 = property on="Bouton Accueil" class="Bool (strict)"("Visible"=TRUE) -> ()  [unwired: 2 in, 2 out]
      n150 = property on="Start acquisition" class="Bool (strict)"("Visible"=TRUE) -> ()  [unwired: 2 in, 2 out]
      n151 = property on="stop" class="Bool (strict)"("Visible"=FALSE) -> ()  [unwired: 2 in, 2 out]
      n152 = property on="Bouton Accueil" class="Bool (strict)"("DisabledEnum"=T2."Enabled" ("Désactivé")) -> ()  [unwired: 2 in, 2 out]
      n153 = property on="sortie d'erreur" class="Clust (strict)"("Value"=errorcluster {"status"=FALSE, "code"=0, "source"=""} ("constante d'erreur")) -> ()  [unwired: 2 in, 2 out]
      n154 = property on="Bouton Accueil" class="Bool (strict)"("DisabledEnum"=T2."Enabled" ("Désactivé")) -> ()  [unwired: 2 in, 2 out]
      n155 = property on="Bouton Accueil" class="Bool (strict)"("Value"=FALSE ("Bouton Accueil")) -> ()  [unwired: 2 in, 2 out]
      n156 = property on="Start acquisition" class="Bool (strict)"("Value"=FALSE) -> ()  [unwired: 2 in, 2 out]
      n157 = property on="stop" class="Bool (strict)"("Value"=FALSE ("stop")) -> ()  [unwired: 2 in, 2 out]
      n158 = property on="Scale (Watt or Joule) (Energie UV)" class="MDér (strict)"("DisabledEnum"=T2."Disabled and Grayed Out" ("Désactivé")) -> ()  [unwired: 2 in, 2 out]
      n159 = property on="Scale (Watt or Joule) (Energie UV)" class="MDér (strict)"("DisabledEnum"=T2."Disabled and Grayed Out" ("Désactivé")) -> ()  [unwired: 2 in, 2 out]
      n160 = property on="Scale (Watt or Joule) (Puissance depolar)" class="MDér (strict)"("DisabledEnum"=T2."Disabled and Grayed Out" ("Désactivé")) -> ()  [unwired: 2 in, 2 out]
      n161 = property on="Scale (Watt or Joule) (Puissance depolar)" class="MDér (strict)"("DisabledEnum"=T2."Disabled and Grayed Out" ("Désactivé")) -> ()  [unwired: 2 in, 2 out]
      n162 = property on="Scale (Watt or Joule) (Energie IR)" class="MDér (strict)"("DisabledEnum"=T2."Disabled and Grayed Out" ("Désactivé")) -> ()  [unwired: 2 in, 2 out]
      n163 = property on="Scale (Watt or Joule) (Energie IR)" class="MDér (strict)"("DisabledEnum"=T2."Disabled and Grayed Out" ("Désactivé")) -> ()  [unwired: 2 in, 2 out]
      n164 = property on="Auto Scale (Puissance depolar)" class="Bool (strict)"("Value"=TRUE) -> ()  [unwired: 2 in, 2 out]
      n165 = property on="Auto Scale (Energie UV)" class="Bool (strict)"("Value"=TRUE) -> ()  [unwired: 2 in, 2 out]
      n166 = property on="Auto Scale (Energie IR)" class="Bool (strict)"("Value"=TRUE ("Auto Scale (Energie IR)")) -> ()  [unwired: 2 in, 2 out]
      "Energie IR mean" <- 0.0 ("mean 3")
      "Energie IR variance" <- 0.0 ("rms value 3")
      "Energie IR max" <- 0.0 ("valeur max 3")
      "Energie IR min" <- 0.0 ("valeur min 3")
      "Energie IR value" <- 0.0 ("Numérique 3")
      "Energie IR graph" <- 0.0 ("Graphe déroulant 3")
      "Puissance depolar value" <- 0.0 ("Numérique 2")
      "Puissance depolar graph" <- 0.0 ("Graphe déroulant 2")
      "Puissance depolar mean" <- 0.0 ("mean 2")
      "Puissance depolar variance" <- 0.0 ("rms value 2")
      "Puissance depolar max" <- 0.0 ("valeur max 2")
      "Puissance depolar min" <- 0.0 ("valeur min 2")
      "Energie IR table" <- dbl[] [] ("Tableau 3")
      "Energie IR table (1sec)" <- dbl[] [] ("Tableau1 3")
      "Puissance depolar table" <- dbl[] [] ("Tableau1 2")
      "Energie UV value" <- 0.0 ("Numérique 1")
      "Energie UV graph" <- 0.0 ("Graphe déroulant 1")
      "Energie UV table" <- dbl[] [] ("Tableau 1")
      "Energie UV mean" <- 0.0 ("mean 1")
      "Energie UV variance" <- 0.0 ("rms value 1")
      "Energie UV max" <- 0.0 ("valeur max 1")
      "Energie UV min" <- 0.0 ("valeur min 1")
      "Energie UV table(1sec)" <- dbl[] [] ("Tableau1 1")
      "Taux depolar value" <- 0.0 ("Numérique 7")
      "taux depolar graph" <- 0.0 ("Graphe déroulant 4")
      "Puissance depolar table (stats)" <- dbl[][] [] ("Tableau stat 2")
      "Energie IR table (stats)" <- dbl[][] [] ("Tableau stat 3")
      "Energie UV rapport" <- 0.0 ("rapport 1")
      "Puissance depolar rapport" <- 0.0 ("rapport 2")
      "Energie IR rapport" <- 0.0 ("rapport 3")
      "Taux depolar indicator" <- u32 16777222 ("taux depolar")
      "Puissance depolar table (1sec)" <- dbl[] [] ("Tableau1 2")
      "Energie UV table (stats)" <- dbl[][] [] ("Tableau stat 1")
      "timer 1sec" <- FALSE ("timer 1s")
      "timer 12sec" <- FALSE ("timer 12s")
      "index 1sec" <- 0 ("index 1sec")
      "index 12sec" <- 0 ("index 12sec")
      "Chaîne" <- "Energie UV" ("Chaîne")
      "Chaîne 4" <- "Energie UV (mJ)" ("Chaîne 4")
      "Chaîne 2" <- "Puissance depolar" ("Chaîne 2")
      "Chaîne 3" <- "Energie IR" ("Chaîne 3")
      "Chaîne 5" <- "Energie IR (mJ)" ("Chaîne 5")
      "Chaîne 6" <- "Puissance depolar (W)" ("Chaîne 6")
      "Chaîne 7" <- "Taux depolar" ("Chaîne 7")
      "Update" <- ""
      "chaîne de date/heure" <- ""
      "valeur de l'horloge en ms" <- u32 0 ("valeur de l'horloge en ms")
      "Time" <- ""
      "stop?" <- FALSE ("stop?")
      "Tableau Puissance depolar" <- dbl[] [] ("Tableau Puissance depolar")
      "Tableau UV" <- dbl[] []
      "Tableau IR" <- dbl[] [] ("Tableau IR")
      "taille UV" <- 0.0 ("taille(s)")
      "taille Pd" <- 0.0 ("taille(s) 2")
      "taille IR" <- 0.0 ("taille(s) 3")
      "12sec UV" <- FALSE ("12sec UV")
      "12sec Pd" <- FALSE ("12sec Pd")
      "12sec IR" <- FALSE ("12sec IR")
      "stop UV" <- FALSE ("stop UV")
      "stop Pd" <- FALSE ("stop Pd")
      "stop IR" <- FALSE ("stop IR")
    }
    frame #1 {
      # "Processing"
      n167 = property on="error IO" class="Clust (strict)"() -> ("Value"=w284:errorcluster)  [unwired: 2 in, 2 out]
      n168 = case shown="Pas d'erreur" w284 {
        selector: w284 -> [_ w825]
        tunnel: [w291 w825] -> w283
        frame No Error {
          w299 = T3 {enum."Stop", "Data"=0.0}
          w317 = T3 {enum."Stop", "Data"=0.0}
          w349 = T3 {enum."Stop", "Data"=0.0}
          n169 = property on="Energie UV file (stats)" class="Ref (strict)"() -> ("Value"=w334:refnum<file>)  [unwired: 2 in, 2 out]
          n170 = property on="Puissance depolar file (stats)" class="Ref (strict)"() -> ("Value"=w333:refnum<file>)  [unwired: 2 in, 2 out]
          n171 = property on="Energie IR file (stats)" class="Ref (strict)"() -> ("Value"=w332:refnum<file>)  [unwired: 2 in, 2 out]
          n172 = property on="Puissance depolar file (500pts)" class="Ref (strict)" props=["Value"]() -> ()  [unwired: 2 in, 3 out]
          n173 = property on="Puissance depolar file (500pts)" class="Ref (strict)"() -> ("Value"=w286:refnum<file>)  [unwired: 2 in, 2 out]
          n174 = property on="Energie IR file (500pts)" class="Ref (strict)" props=["Value"]() -> ()  [unwired: 2 in, 3 out]
          n175 = property on="Energie IR file (500pts)" class="Ref (strict)"() -> ("Value"=w287:refnum<file>)  [unwired: 2 in, 2 out]
          n176 = property on="Energy UV file (500pts)" class="Ref (strict)"() -> ("Value"=w285:refnum<file>)  [unwired: 2 in, 2 out]
          n177 = while {
            tunnel: w334 -> [w635]
            tunnel: w333 -> [w634]
            tunnel: w332 -> [w633]
            tunnel: w287 -> [w631]
            tunnel: w286 -> [w630]
            tunnel: w285 -> [w629]
            stop <- w632 stop-if-true
            # "actions à réaliser toutes les 12sec"
            n178 = event shown="[0] \"12sec\": Valeur changée" {
              selector: _ -> [_ _]
              dyn-events: _ -> [_ _]
              timeout: _ -> [_ _]
              tunnel: w635 -> [w706 _]
              tunnel: w634 -> [w705 _]
              tunnel: w633 -> [w704 _]
              tunnel: [FALSE TRUE] -> w632
              tunnel: w631 -> [w638 _]
              tunnel: w630 -> [w637 _]
              tunnel: w629 -> [w636 _]
              event "12sec": Value Change {
                w645 = ","
                w649 = ","
                w651 = ","
                w652 = "\t"
                w698 = ","
                n179 = event-data() -> ()  [unwired: 1 in, 6 out]
                n180 = property on="Tableau UV" class="Tabl (strict)"() -> ("Value"=w642:dbl[])  [unwired: 2 in, 2 out]
                n181 = call <vilib>:"Std Deviation and Variance.vi"("X"=w642) -> ("mean"=w677:dbl, "standard deviation"=w676:dbl)  [unwired: 1 in, 1 out]
                n182 = Array Max & Min(array=w642) -> (max value=w675:dbl, min value=w674:dbl)  [unwired: 2 out]
                n183 = Array Size(array=w642) -> (size(s)=w684:i32)
                n184 = property on="Tableau Puissance depolar" class="Tabl (strict)"() -> ("Value"=w643:dbl[])  [unwired: 2 in, 2 out]
                n185 = To Double Precision Float(number=w684) -> (double precision float=w662:dbl)
                n186 = Get Date/Time In Seconds() -> (seconds since 1Jan1904=w696:timestamp)
                n187 = Format Date/Time String(time format string (%c)="%d-%m-%Y-%H:%M:%S%3u", seconds (now)=w696) -> (date/time string=w699:string)  [unwired: 1 in]
                n188 = Divide(x=w676, y=w677) -> (x/y=w688:dbl)
                n189 = property on="taille UV" class="NumNb (strict)"("Value"=w662) -> ()  [unwired: 2 in, 2 out]
                n190 = property on="Energie UV mean" class="NumNb (strict)"("Value"=w677) -> ()  [unwired: 2 in, 2 out]
                n191 = property on="Energie UV variance" class="NumNb (strict)"("Value"=w676) -> ()  [unwired: 2 in, 2 out]
                n192 = property on="Energie UV max" class="NumNb (strict)"("Value"=w675) -> ()  [unwired: 2 in, 2 out]
                n193 = property on="Energie UV min" class="NumNb (strict)"("Value"=w674) -> ()  [unwired: 2 in, 2 out]
                n194 = Multiply(x=w688, y=100.0) -> (x*y=w673:dbl)
                n195 = property on="valeur de l'horloge en ms" class="NumNb (strict)"() -> ("Value"=w700:u32)  [unwired: 2 in, 2 out]
                n196 = Tick Count (ms)() -> (millisecond timer value=w701:u32)
                n197 = property on="Energie UV rapport" class="NumNb (strict)"("Value"=w673) -> ()  [unwired: 2 in, 2 out]
                n198 = Build Array(w677, w676, w675, w674, w673) -> (w650:dbl[])
                n199 = call <vilib>:"Std Deviation and Variance.vi"("X"=w643) -> ("mean"=w668:dbl, "standard deviation"=w669:dbl)  [unwired: 1 in, 1 out]
                n200 = Array Max & Min(array=w643) -> (max value=w670:dbl, min value=w671:dbl)  [unwired: 2 out]
                n201 = Array Size(array=w643) -> (size(s)=w683:i32)
                n202 = property on="Tableau IR" class="Tabl (strict)"() -> ("Value"=w644:dbl[])  [unwired: 2 in, 2 out]
                n203 = To Double Precision Float(number=w683) -> (double precision float=w661:dbl)
                n204 = Divide(x=w669, y=w668) -> (x/y=w686:dbl)
                n205 = property on="taille Pd" class="NumNb (strict)"("Value"=w661) -> ()  [unwired: 2 in, 2 out]
                n206 = Subtract(x=w701, y=w700) -> (x-y=w702:u32)
                n207 = property on="Puissance depolar mean" class="NumNb (strict)"("Value"=w668) -> ()  [unwired: 2 in, 2 out]
                n208 = property on="Puissance depolar variance" class="NumNb (strict)"("Value"=w669) -> ()  [unwired: 2 in, 2 out]
                n209 = property on="Puissance depolar max" class="NumNb (strict)"("Value"=w670) -> ()  [unwired: 2 in, 2 out]
                n210 = property on="Puissance depolar min" class="NumNb (strict)"("Value"=w671) -> ()  [unwired: 2 in, 2 out]
                n211 = Number To Decimal String(number=w702) -> (decimal integer string=w703:string)  [unwired: 1 in]
                n212 = Multiply(x=w686, y=100.0) -> (x*y=w672:dbl)
                n213 = Build Array(w668, w669, w670, w671, w672) -> (w682:dbl[])
                n214 = Concatenate Strings(w699, w698, w703, w698) -> (w689:string)
                n215 = property on="Puissance depolar rapport" class="NumNb (strict)"("Value"=w672) -> ()  [unwired: 2 in, 2 out]
                n216 = call <vilib>:"Std Deviation and Variance.vi"("X"=w644) -> ("mean"=w663:dbl, "standard deviation"=w664:dbl)  [unwired: 1 in, 1 out]
                n217 = Array Max & Min(array=w644) -> (max value=w665:dbl, min value=w666:dbl)  [unwired: 2 out]
                n218 = Array Size(array=w644) -> (size(s)=w681:i32)
                n219 = To Double Precision Float(number=w681) -> (double precision float=w660:dbl)
                n220 = Divide(x=w664, y=w663) -> (x/y=w679:dbl)
                n221 = property on="taille IR" class="NumNb (strict)"("Value"=w660) -> ()  [unwired: 2 in, 2 out]
                n222 = Multiply(x=w679, y=100.0) -> (x*y=w667:dbl)
                n223 = property on="Energie IR mean" class="NumNb (strict)"("Value"=w663) -> ()  [unwired: 2 in, 2 out]
                n224 = property on="Energie IR variance" class="NumNb (strict)"("Value"=w664) -> ()  [unwired: 2 in, 2 out]
                n225 = property on="Energie IR max" class="NumNb (strict)"("Value"=w665) -> ()  [unwired: 2 in, 2 out]
                n226 = property on="Energie IR min" class="NumNb (strict)"("Value"=w666) -> ()  [unwired: 2 in, 2 out]
                n227 = Build Array(w663, w664, w665, w666, w667) -> (w678:dbl[])
                n228 = property on="Energie IR rapport" class="NumNb (strict)"("Value"=w667) -> ()  [unwired: 2 in, 2 out]
                n229 = Array To Spreadsheet String(delimiter (Tab)=w649, array=w650, 3:"%f" ("chaîne de format")) -> (spreadsheet string=w658:string)
                n230 = Array To Spreadsheet String(delimiter (Tab)=w649, array=w682, 3:"%f" ("chaîne de format")) -> (spreadsheet string=w656:string)
                n231 = Array To Spreadsheet String(delimiter (Tab)=w649, array=w678, 3:"%f" ("chaîne de format")) -> (spreadsheet string=w655:string)
                n232 = Array To Spreadsheet String(delimiter (Tab)=w645, array=w642, 3:"%f" ("chaîne de format")) -> (spreadsheet string=w641:string)
                n233 = Array To Spreadsheet String(delimiter (Tab)=w645, array=w644, 3:"%f" ("chaîne de format")) -> (spreadsheet string=w639:string)
                n234 = Array To Spreadsheet String(delimiter (Tab)=w645, array=w643, 3:"%f" ("chaîne de format")) -> (spreadsheet string=w640:string)
                n235 = Write to Text File(file (use dialog)=w636, text=w641) -> ()  [unwired: 2 in, 3 out]
                n236 = Write to Text File(file (use dialog)=w637, text=w640) -> ()  [unwired: 2 in, 3 out]
                n237 = Write to Text File(file (use dialog)=w638, text=w639) -> ()  [unwired: 2 in, 3 out]
                n238 = Search and Replace String(input string=w655, search string=w652, replace string=w651) -> (result string=w654:string)  [unwired: 5 in, 3 out]
                n239 = Search and Replace String(input string=w658, search string=w652, replace string=w651) -> (result string=w657:string)  [unwired: 5 in, 3 out]
                n240 = Search and Replace String(input string=w656, search string=w652, replace string=w651) -> (result string=w653:string)  [unwired: 5 in, 3 out]
                n241 = Concatenate Strings(w689, w657) -> (w694:string)
                n242 = Concatenate Strings(w689, w653) -> (w692:string)
                n243 = Concatenate Strings(w689, w654) -> (w690:string)
                n244 = Write to Text File(file (use dialog)=w706, text=w694) -> ()  [unwired: 2 in, 3 out]
                n245 = Write to Text File(file (use dialog)=w705, text=w692) -> ()  [unwired: 2 in, 3 out]
                n246 = Write to Text File(file (use dialog)=w704, text=w690) -> ()  [unwired: 2 in, 3 out]
              }
              event "stop": Value Change {
                n247 = event-data() -> ()  [unwired: 1 in, 6 out]
                n248 = property on="stop UV" class="Bool (strict)"("Val(Sgnl)"=TRUE ("Valeur (Signalisation)")) -> ()  [unwired: 2 in, 2 out]
                n249 = property on="stop Pd" class="Bool (strict)"("Val(Sgnl)"=TRUE ("Valeur (Signalisation)")) -> ()  [unwired: 2 in, 2 out]
                n250 = property on="stop IR" class="Bool (strict)"("Val(Sgnl)"=TRUE ("Valeur (Signalisation)")) -> ()  [unwired: 2 in, 2 out]
              }
            }
          }
          n251 = Obtain Queue(name (unnamed)="Energie UV" ("nom (aucun)"), element data type=w349) -> (queue out=w350:refnum<queue>, error out=w351:errorcluster)  [unwired: 3 in, 1 out]
          n252 = property on="COM Port table" class="Tabl (strict)"() -> ("Value"=w343:refnum<visa-resource-name>[])  [unwired: 2 in, 2 out]
          n253 = Bundle(cluster=w349, enum16{"Init", "Read", "Stop", "12sec"}."Init") -> (w352:T3)  [unwired: 1 in]
          n254 = Enqueue Element At Opposite End(queue=w350, element=w352, error in (no error)=w351) -> (queue out=w348:refnum<queue>, error out=w328:errorcluster)  [unwired: 1 in, 1 out]
          n255 = Index Array(array=w343, index=0 ("indice")) -> (element=w339:refnum<visa-resource-name>)
          n256 = call "Send Continuous Value (SubVI).vi"("entrée d'erreur"=w328, "Refnum VISA en entrée"=w339) -> ("sortie d'erreur"=w338:errorcluster, "Refnum VISA en sortie"=w337:refnum<visa-resource-name>)
          n257 = while {
            tunnel: w349 -> [w363]
            shift-right: [w362] -> w330
            shift-left: w328 -> [w361]
            shift-right: [w360] -> _
            shift-left: w348 -> [w364]
            shift-right: [w356] -> w329
            shift-left: w338 -> [w357]
            shift-right: [w354] -> _
            shift-left: w337 -> [w358]
            stop <- w359 stop-if-true
            n258 = event shown="[2] \"stop UV\": Valeur changée" {
              selector: _ -> [_ _ _]
              dyn-events: _ -> [_ _ _]
              timeout: 1 -> [_ _ _]
              tunnel: w364 -> [w380 w397 w409]
              tunnel: w363 -> [w379 w396 w412]
              tunnel: [w375 w392 w407] -> w362
              tunnel: w361 -> [w377 w394 w410]
              tunnel: [w376 w393 w411] -> w360
              tunnel: [w374 w391 w406] -> w359
              tunnel: w358 -> [w365 w387 w402]
              tunnel: w357 -> [w366 w381 w401]
              tunnel: [w369 w385 w400] -> w356
              tunnel: [w368 w384 w399] -> w354
              event Timeout {
                n259 = event-data() -> ()  [unwired: 1 in, 1 out]
                n260 = call "Read Continuous Value (SubVI).vi"("error in"=w366, "VISA Refnum in"=w365) -> ("error out"=w369:errorcluster, "nombre"=w370:dbl, "VISA Refnum out"=w368:refnum<visa-resource-name>)  [unwired: 6 in, 1 out]
                n261 = Bundle(cluster=w379, enum16{"Init", "Read", "Stop", "12sec"}."Read", "Data"=w370) -> (w378:T3)
                n262 = Enqueue Element(queue=w380, element=w378, error in (no error)=w377) -> (queue out=w376:refnum<queue>, error out=w375:errorcluster)  [unwired: 1 in, 1 out]
                n263 = Unbundle By Name(w375) -> ("status"=w372:bool)
                n264 = Unbundle By Name(w369) -> ("status"=w371:bool)
                n265 = Compound Arithmetic op=OR ("Opérateur arithmétique")(w371, w372, FALSE) -> (w374:bool)
              }
              event "12sec UV": Value Change {
                n266 = event-data() -> ()  [unwired: 1 in, 1 out]
                n267 = call "Read Continuous Value (SubVI).vi"("error in"=w381, "VISA Refnum in"=w387) -> ("error out"=w385:errorcluster, "nombre"=w386:dbl, "VISA Refnum out"=w384:refnum<visa-resource-name>)  [unwired: 6 in, 1 out]
                n268 = Bundle(cluster=w396, enum16{"Init", "Read", "Stop", "12sec"}."12sec", "Data"=w386) -> (w395:T3)
                n269 = Enqueue Element(queue=w397, element=w395, error in (no error)=w394) -> (queue out=w393:refnum<queue>, error out=w392:errorcluster)  [unwired: 1 in, 1 out]
                n270 = Unbundle By Name(w392) -> ("status"=w389:bool)
                n271 = Unbundle By Name(w385) -> ("status"=w388:bool)
                n272 = property on="12sec UV" class="Bool (strict)"("Value"=FALSE ("12sec UV")) -> ()  [unwired: 2 in, 2 out]
                n273 = Compound Arithmetic op=OR ("Opérateur arithmétique")(w388, w389, FALSE) -> (w391:bool)
              }
              event "stop UV": Value Change {
                n274 = event-data() -> ()  [unwired: 1 in, 6 out]
                n275 = Bundle(cluster=w412, enum16{"Init", "Read", "Stop", "12sec"}."Stop") -> (w408:T3)  [unwired: 1 in]
                n276 = Enqueue Element(queue=w409, element=w408, error in (no error)=w410) -> (queue out=w411:refnum<queue>, error out=w407:errorcluster)  [unwired: 1 in, 1 out]
                n277 = call "Stop Continuous Value (SubVI).vi"("entrée d'erreur"=w401, "Refnum VISA en entrée"=w402) -> ("sortie d'erreur"=w400:errorcluster, "Refnum VISA en sortie"=w399:refnum<visa-resource-name>)
                n278 = Unbundle By Name(w407) -> ("status"=w404:bool)
                n279 = Unbundle By Name(w400) -> ("status"=w403:bool)
                n280 = Compound Arithmetic op=OR ("Opérateur arithmétique")(w403, w404, TRUE) -> (w406:bool)
              }
            }
          }
          n281 = while {
            shift-right: [w783] -> w347
            shift-left: w328 -> [w789]
            shift-right: [w782] -> w346
            shift-left: w348 -> [w784]
            shift-right: [w779] -> _
            shift-left: _ -> [w780]
            stop <- w781 stop-if-true
            n282 = Dequeue Element(queue=w784, error in (no error)=w789) -> (queue out=w785:refnum<queue>, element=w788:T3, error out=w786:errorcluster)  [unwired: 1 in, 1 out]
            n283 = Unbundle(w788) -> (w787:enum16{"Init", "Read", "Stop", "12sec"}, "Data"=w778:dbl)
            n284 = case shown="\"12sec\"" w787 {
              tunnel: w780 -> [_ w797 w808 w819]
              tunnel: w778 -> [_ w795 w806 _]
              tunnel: w786 -> [w793 w800 w813 w824]
              tunnel: w785 -> [w791 w798 w811 w823]
              tunnel: [w793 w800 w813 w822] -> w783
              tunnel: [FALSE FALSE FALSE TRUE] -> w781
              tunnel: [w791 w798 w811 w820] -> w782
              tunnel: [dbl[] [] w796 dbl[] [] w819] -> w779
              frame "Init", Default {
              }
              frame "Read" {
                n285 = for {
                  N: 1 -> [_]
                  tunnel: w797 -> [w805]
                  tunnel: [w804] -> w796 if=w801
                  tunnel: w795 -> [w803]
                  n286 = Equal To 0?(x=w803) -> (x = 0?=w802:bool)
                  n287 = Insert Into Array(array=w805, new element=w803) -> (w804:dbl[])  [unwired: 1 in]
                  n288 = Not(x=w802) -> (.not. x?=w801:bool)
                }
                n289 = property on="Tableau UV" class="Tabl (strict)"("Value"=w796) -> ()  [unwired: 2 in, 2 out]
              }
              frame "12sec" {
                n290 = for {
                  N: 1 -> [_]
                  tunnel: w808 -> [w818]
                  tunnel: [w817] -> w807 if=w814
                  tunnel: w806 -> [w816]
                  n291 = Equal To 0?(x=w816) -> (x = 0?=w815:bool)
                  n292 = Insert Into Array(array=w818, new element=w816) -> (w817:dbl[])  [unwired: 1 in]
                  n293 = Not(x=w815) -> (.not. x?=w814:bool)
                }
                n294 = property on="Tableau UV" class="Tabl (strict)"("Value"=w807) -> ()  [unwired: 2 in, 2 out]
              }
              frame "Stop" {
                n295 = Flush Queue(queue=w823, error in (no error)=w824) -> (queue out=w820:refnum<queue>, error out=w822:errorcluster)  [unwired: 1 out]
              }
            }
          }
          n296 = Release Queue(queue=w346, error in (no error)=w347) -> (error out=w331:errorcluster)  [unwired: 1 in, 2 out]
          n297 = Merge Errors(w329, w330, w331) -> (w292:errorcluster)
          n298 = Obtain Queue(name (unnamed)="Puissance depolar" ("nom (aucun)"), element data type=w317) -> (queue out=w316:refnum<queue>, error out=w315:errorcluster)  [unwired: 3 in, 1 out]
          n299 = property on="COM Port table" class="Tabl (strict)"() -> ("Value"=w322:refnum<visa-resource-name>[])  [unwired: 2 in, 2 out]
          n300 = Bundle(cluster=w317, enum16{"Init", "Read", "Stop", "12sec"}."Init") -> (w314:T3)  [unwired: 1 in]
          n301 = while {
            shift-right: [w714] -> _
            shift-left: 0.0 -> [w713]
            stop <- w716 stop-if-true
            # "Timer"
            n302 = Equal?(x=w713, y=11.0) -> (x = y?=w712:bool)
            n303 = case shown="Vrai" w712 {
              selector: w712 -> [w720 _]
              tunnel: [0.0 w723] -> w714
              tunnel: w713 -> [_ w722]
              frame True {
                n304 = property on="12sec" class="Bool (strict)"("Val(Sgnl)"=w720) -> ()  [unwired: 2 in, 2 out]
                n305 = property on="12sec UV" class="Bool (strict)"("Val(Sgnl)"=TRUE ("12sec UV")) -> ()  [unwired: 2 in, 2 out]
                n306 = property on="12sec Pd" class="Bool (strict)"("Val(Sgnl)"=TRUE ("12sec Pd")) -> ()  [unwired: 2 in, 2 out]
                n307 = property on="12sec IR" class="Bool (strict)"("Val(Sgnl)"=TRUE ("12sec IR")) -> ()  [unwired: 2 in, 2 out]
              }
              frame False {
                n308 = Increment(x=w722) -> (x+1=w723:dbl)
              }
            }
            n309 = Wait Until Next ms Multiple(millisecond multiple=u32 1000 ("attente (ms)")) -> ()  [unwired: 1 out]
            n310 = property on="stop" class="Bool (strict)"() -> ("Value"=w716:bool)  [unwired: 2 in, 2 out]
          }
          n311 = Enqueue Element At Opposite End(queue=w316, element=w314, error in (no error)=w315) -> (queue out=w318:refnum<queue>, error out=w327:errorcluster)  [unwired: 1 in, 1 out]
          n312 = Index Array(array=w322, index=1 ("indice")) -> (element=w289:refnum<visa-resource-name>)
          n313 = call "Send Continuous Value (SubVI).vi"("entrée d'erreur"=w327, "Refnum VISA en entrée"=w289) -> ("sortie d'erreur"=w290:errorcluster, "Refnum VISA en sortie"=w288:refnum<visa-resource-name>)
          n314 = while {
            tunnel: w317 -> [w422]
            shift-right: [w421] -> w325
            shift-left: w327 -> [w420]
            shift-right: [w419] -> _
            shift-left: w318 -> [w423]
            shift-right: [w415] -> w326
            shift-left: w290 -> [w416]
            shift-right: [w413] -> _
            shift-left: w288 -> [w417]
            stop <- w418 stop-if-true
            n315 = event shown="[0] Timeout" {
              selector: _ -> [_ _ _]
              dyn-events: _ -> [_ _ _]
              timeout: 100 -> [_ _ _]
              tunnel: w423 -> [w441 w460 w472]
              tunnel: w422 -> [w440 w459 w475]
              tunnel: [w436 w455 w470] -> w421
              tunnel: w420 -> [w438 w457 w473]
              tunnel: [w437 w456 w474] -> w419
              tunnel: [w435 w454 w469] -> w418
              tunnel: w417 -> [w428 w444 w465]
              tunnel: w416 -> [w426 w446 w462]
              tunnel: [w425 w445 w461] -> w415
              tunnel: [w427 w443 w463] -> w413
              event Timeout {
                n316 = event-data() -> ()  [unwired: 1 in, 1 out]
                n317 = call "Read Continuous Value (SubVI).vi"("error in"=w426, "VISA Refnum in"=w428) -> ("error out"=w425:errorcluster, "nombre"=w424:dbl, "VISA Refnum out"=w427:refnum<visa-resource-name>)  [unwired: 6 in, 1 out]
                n318 = Divide(x=w424, y=1000.0) -> (x/y=w430:dbl)
                n319 = Bundle(cluster=w440, enum16{"Init", "Read", "Stop", "12sec"}."Read", "Data"=w430) -> (w439:T3)
                n320 = Enqueue Element(queue=w441, element=w439, error in (no error)=w438) -> (queue out=w437:refnum<queue>, error out=w436:errorcluster)  [unwired: 1 in, 1 out]
                n321 = Unbundle By Name(w436) -> ("status"=w433:bool)
                n322 = Unbundle By Name(w425) -> ("status"=w432:bool)
                n323 = Compound Arithmetic op=OR ("Opérateur arithmétique")(w432, w433, FALSE) -> (w435:bool)
              }
              event "12sec Pd": Value Change {
                n324 = event-data() -> ()  [unwired: 1 in, 1 out]
                n325 = call "Read Continuous Value (SubVI).vi"("error in"=w446, "VISA Refnum in"=w444) -> ("error out"=w445:errorcluster, "nombre"=w442:dbl, "VISA Refnum out"=w443:refnum<visa-resource-name>)  [unwired: 6 in, 1 out]
                n326 = Divide(x=w442, y=1000.0) -> (x/y=w449:dbl)
                n327 = Bundle(cluster=w459, enum16{"Init", "Read", "Stop", "12sec"}."12sec", "Data"=w449) -> (w458:T3)
                n328 = property on="12sec Pd" class="Bool (strict)"("Value"=FALSE ("12sec Pd")) -> ()  [unwired: 2 in, 2 out]
                n329 = Enqueue Element(queue=w460, element=w458, error in (no error)=w457) -> (queue out=w456:refnum<queue>, error out=w455:errorcluster)  [unwired: 1 in, 1 out]
                n330 = Unbundle By Name(w455) -> ("status"=w452:bool)
                n331 = Unbundle By Name(w445) -> ("status"=w451:bool)
                n332 = Compound Arithmetic op=OR ("Opérateur arithmétique")(w451, w452, FALSE) -> (w454:bool)
              }
              event "stop Pd": Value Change {
                n333 = event-data() -> ()  [unwired: 1 in, 6 out]
                n334 = Bundle(cluster=w475, enum16{"Init", "Read", "Stop", "12sec"}."Stop") -> (w471:T3)  [unwired: 1 in]
                n335 = Enqueue Element(queue=w472, element=w471, error in (no error)=w473) -> (queue out=w474:refnum<queue>, error out=w470:errorcluster)  [unwired: 1 in, 1 out]
                n336 = call "Stop Continuous Value (SubVI).vi"("entrée d'erreur"=w462, "Refnum VISA en entrée"=w465) -> ("sortie d'erreur"=w461:errorcluster, "Refnum VISA en sortie"=w463:refnum<visa-resource-name>)
                n337 = Unbundle By Name(w470) -> ("status"=w467:bool)
                n338 = Unbundle By Name(w461) -> ("status"=w466:bool)
                n339 = Compound Arithmetic op=OR ("Opérateur arithmétique")(w466, w467, TRUE) -> (w469:bool)
              }
            }
          }
          n340 = while {
            shift-right: [w586] -> w319
            shift-left: w327 -> [w593]
            shift-right: [w585] -> w320
            shift-left: w318 -> [w587]
            shift-right: [w582] -> _
            shift-left: _ -> [w583]
            stop <- w584 stop-if-true
            n341 = Dequeue Element(queue=w587, error in (no error)=w593) -> (queue out=w588:refnum<queue>, element=w592:T3, error out=w589:errorcluster)  [unwired: 1 in, 1 out]
            n342 = Unbundle(w592) -> (w591:enum16{"Init", "Read", "Stop", "12sec"}, "Data"=w590:dbl)
            n343 = case shown="\"Read\"" w591 {
              tunnel: w583 -> [_ w600 w612 w623]
              tunnel: w590 -> [_ w599 w611 _]
              tunnel: w589 -> [w597 w604 w617 w628]
              tunnel: w588 -> [w595 w602 w615 w627]
              tunnel: [w597 w604 w617 w626] -> w586
              tunnel: [FALSE FALSE FALSE TRUE] -> w584
              tunnel: [w595 w602 w615 w624] -> w585
              tunnel: [dbl[] [] w598 dbl[] [] w623] -> w582
              frame "Init", Default {
              }
              frame "Read" {
                n344 = for {
                  N: 1 -> [_]
                  tunnel: [w609] -> w598 if=w607
                  tunnel: w600 -> [w606]
                  tunnel: w599 -> [w605]
                  n345 = Equal To 0?(x=w605) -> (x = 0?=w608:bool)
                  n346 = Insert Into Array(array=w606, new element=w605) -> (w609:dbl[])  [unwired: 1 in]
                  n347 = Not(x=w608) -> (.not. x?=w607:bool)
                }
                n348 = property on="Tableau Puissance depolar" class="Tabl (strict)"("Value"=w598) -> ()  [unwired: 2 in, 2 out]
              }
              frame "12sec" {
                n349 = for {
                  N: 1 -> [_]
                  tunnel: w612 -> [w622]
                  tunnel: [w621] -> w610 if=w618
                  tunnel: w611 -> [w620]
                  n350 = Equal To 0?(x=w620) -> (x = 0?=w619:bool)
                  n351 = Insert Into Array(array=w622, new element=w620) -> (w621:dbl[])  [unwired: 1 in]
                  n352 = Not(x=w619) -> (.not. x?=w618:bool)
                }
                n353 = property on="Tableau Puissance depolar" class="Tabl (strict)"("Value"=w610) -> ()  [unwired: 2 in, 2 out]
              }
              frame "Stop" {
                n354 = Flush Queue(queue=w627, error in (no error)=w628) -> (queue out=w624:refnum<queue>, error out=w626:errorcluster)  [unwired: 1 out]
              }
            }
          }
          n355 = property on="Update" class="Ch"("Value"="Data acquisition" ("Étiquette.Texte")) -> ()  [unwired: 2 in, 2 out]
          n356 = property on="Energie UV file (1sec)" class="Ref (strict)"() -> ("Value"=w340:refnum<file>)  [unwired: 2 in, 2 out]
          n357 = property on="Puissance depolar file (1sec)" class="Ref (strict)"() -> ("Value"=w342:refnum<file>)  [unwired: 2 in, 2 out]
          n358 = property on="Energie IR file (1sec)" class="Ref (strict)"() -> ("Value"=w341:refnum<file>)  [unwired: 2 in, 2 out]
          n359 = while {
            tunnel: w342 -> [w751]
            tunnel: w341 -> [w740]
            tunnel: w340 -> [w739]
            stop <- w774 stop-if-true
            w747 = ","
            w748 = "\r\n"
            # "actions à réaliser toutes les 1sec"
            n360 = property on="Tableau Puissance depolar" class="Tabl (strict)"() -> ("Value"=w735:dbl[])  [unwired: 2 in, 2 out]
            n361 = property on="Tableau IR" class="Tabl (strict)"() -> ("Value"=w730:dbl[])  [unwired: 2 in, 2 out]
            n362 = property on="Tableau UV" class="Tabl (strict)"() -> ("Value"=w732:dbl[])  [unwired: 2 in, 2 out]
            n363 = Array Size(array=w732) -> (size(s)=w729:i32)
            n364 = Array Size(array=w735) -> (size(s)=w727:i32)
            n365 = Subtract(x=w729, y=10) -> (x-y=w738:i32)
            n366 = Array Size(array=w730) -> (size(s)=w725:i32)
            n367 = Subtract(x=w727, y=1) -> (x-y=w737:i32)
            n368 = Subtract(x=w725, y=10) -> (x-y=w736:i32)
            n369 = Index Array(array=w732, index=w738) -> (element=w731:dbl)
            n370 = Get Date/Time In Seconds() -> (seconds since 1Jan1904=w750:timestamp)
            n371 = Format Date/Time String(time format string (%c)="%d-%m-%Y-%H:%M:%S%3u", seconds (now)=w750) -> (date/time string=w746:string)  [unwired: 1 in]
            n372 = Index Array(array=w735, index=w737) -> (element=w733:dbl)
            n373 = Index Array(array=w730, index=w736) -> (element=w734:dbl)
            n374 = property on="Energie UV value" class="NumNb (strict)"("Value"=w731) -> ()  [unwired: 2 in, 2 out]
            n375 = property on="Energie UV graph" class="GraphDér (strict)"("Value"=w731) -> ()  [unwired: 2 in, 2 out]
            n376 = property on="valeur de l'horloge en ms" class="NumNb (strict)"() -> ("Value"=w745:u32)  [unwired: 2 in, 2 out]
            n377 = Tick Count (ms)() -> (millisecond timer value=w744:u32)
            n378 = property on="Puissance depolar graph" class="GraphDér (strict)"("Value"=w733) -> ()  [unwired: 2 in, 2 out]
            n379 = property on="Puissance depolar value" class="NumNb (strict)"("Value"=w733) -> ()  [unwired: 2 in, 2 out]
            n380 = Number To Fractional String(number=w731) -> (F-format string=w756:string)  [unwired: 3 in]
            n381 = property on="Energie IR value" class="NumNb (strict)"("Value"=w734) -> ()  [unwired: 2 in, 2 out]
            n382 = property on="Energie IR graph" class="GraphDér (strict)"("Value"=w734) -> ()  [unwired: 2 in, 2 out]
            n383 = Subtract(x=w744, y=w745) -> (x-y=w743:u32)
            n384 = Number To Decimal String(number=w743) -> (decimal integer string=w742:string)  [unwired: 1 in]
            n385 = Concatenate Strings(w746, w747, w742, w747) -> (w741:string)
            n386 = Concatenate Strings(w741, w756, w748) -> (w757:string)
            n387 = Write to Text File(file (use dialog)=w739, text=w757) -> ()  [unwired: 2 in, 3 out]
            n388 = Number To Fractional String(number=w733) -> (F-format string=w754:string)  [unwired: 3 in]
            n389 = property on="Puissance depolar value" class="NumNb (strict)"() -> ("Value"=w770:dbl)  [unwired: 2 in, 2 out]
            n390 = property on="Energie IR value" class="NumNb (strict)"() -> ("Value"=w760:dbl)  [unwired: 2 in, 2 out]
            n391 = Divide(x=w760, y=1000.0) -> (x/y=w758:dbl)
            n392 = Number To Fractional String(number=w734) -> (F-format string=w752:string)  [unwired: 3 in]
            n393 = Concatenate Strings(w741, w754, w748) -> (w755:string)
            n394 = Multiply(x=w758, y=500.0) -> (x*y=w773:dbl)
            n395 = Write to Text File(file (use dialog)=w751, text=w755) -> ()  [unwired: 2 in, 3 out]
            n396 = Concatenate Strings(w741, w752, w748) -> (w753:string)
            n397 = Add(x=w770, y=w773) -> (x+y=w772:dbl)
            n398 = Write to Text File(file (use dialog)=w740, text=w753) -> ()  [unwired: 2 in, 3 out]
            n399 = Divide(x=w770, y=w772) -> (x/y=w769:dbl)
            n400 = Multiply(x=w769, y=100.0) -> (x*y=w764:dbl)
            n401 = property on="Taux depolar value" class="NumNb (strict)"("Value"=w764) -> ()  [unwired: 2 in, 2 out]
            n402 = property on="taux depolar graph" class="GraphDér (strict)"("Value"=w764) -> ()  [unwired: 2 in, 2 out]
            n403 = Greater Or Equal?(x=w764, y=11.0) -> (x >= y?=w762:bool)
            n404 = Less Or Equal?(x=w764, y=9.0) -> (x <= y?=w765:bool)
            n405 = And(x=w765, y=w762) -> (x .and. y?=w763:bool)
            n406 = case shown="Vrai" w765 {
              frame False {
              }
              frame True {
                n407 = property on="Taux depolar indicator" class="BteCoul"("Value"=u32 6618880 ("Boîte de couleur")) -> ()  [unwired: 2 in, 2 out]
              }
            }
            n408 = case shown="Vrai" w763 {
              frame False {
              }
              frame True {
                n409 = property on="Taux depolar indicator" class="BteCoul"("Value"=u32 16755474 ("Boîte de couleur")) -> ()  [unwired: 2 in, 2 out]
              }
            }
            n410 = case shown="Vrai" w762 {
              frame False {
              }
              frame True {
                n411 = property on="Taux depolar indicator" class="BteCoul"("Value"=u32 16711680 ("Boîte de couleur")) -> ()  [unwired: 2 in, 2 out]
              }
            }
            n412 = property on="stop" class="Bool (strict)"() -> ("Value"=w774:bool)  [unwired: 2 in, 2 out]
            n413 = Wait Until Next ms Multiple(millisecond multiple=u32 1000 ("attente (ms)")) -> ()  [unwired: 1 out]
          }
          n414 = Release Queue(queue=w320, error in (no error)=w319) -> (error out=w324:errorcluster)  [unwired: 1 in, 2 out]
          n415 = Merge Errors(w326, w325, w324) -> (w293:errorcluster)
          n416 = Obtain Queue(name (unnamed)="Energie IR" ("nom (aucun)"), element data type=w299) -> (queue out=w298:refnum<queue>, error out=w297:errorcluster)  [unwired: 3 in, 1 out]
          n417 = property on="COM Port table" class="Tabl (strict)"() -> ("Value"=w304:refnum<visa-resource-name>[])  [unwired: 2 in, 2 out]
          n418 = Bundle(cluster=w299, enum16{"Init", "Read", "Stop", "12sec"}."Init") -> (w296:T3)  [unwired: 1 in]
          n419 = Enqueue Element At Opposite End(queue=w298, element=w296, error in (no error)=w297) -> (queue out=w300:refnum<queue>, error out=w312:errorcluster)  [unwired: 1 in, 1 out]
          n420 = Index Array(array=w304, index=2 ("indice")) -> (element=w305:refnum<visa-resource-name>)
          n421 = call "Send Continuous Value (SubVI).vi"("entrée d'erreur"=w312, "Refnum VISA en entrée"=w305) -> ("sortie d'erreur"=w306:errorcluster, "Refnum VISA en sortie"=w307:refnum<visa-resource-name>)
          n422 = while {
            tunnel: w299 -> [w485]
            shift-right: [w484] -> w310
            shift-left: w312 -> [w483]
            shift-right: [w482] -> _
            shift-left: w300 -> [w486]
            shift-right: [w478] -> w311
            shift-left: w306 -> [w479]
            shift-right: [w476] -> _
            shift-left: w307 -> [w480]
            stop <- w481 stop-if-true
            n423 = event shown="[0] Timeout" {
              selector: _ -> [_ _ _]
              dyn-events: _ -> [_ _ _]
              timeout: 1 -> [_ _ _]
              tunnel: w486 -> [w502 w519 w531]
              tunnel: w485 -> [w501 w518 w534]
              tunnel: [w497 w514 w529] -> w484
              tunnel: w483 -> [w499 w516 w532]
              tunnel: [w498 w515 w533] -> w482
              tunnel: [w496 w513 w528] -> w481
              tunnel: w480 -> [w487 w509 w524]
              tunnel: w479 -> [w488 w503 w523]
              tunnel: [w491 w507 w522] -> w478
              tunnel: [w490 w506 w521] -> w476
              event Timeout {
                n424 = event-data() -> ()  [unwired: 1 in, 1 out]
                n425 = call "Read Continuous Value (SubVI).vi"("error in"=w488, "VISA Refnum in"=w487) -> ("error out"=w491:errorcluster, "nombre"=w492:dbl, "VISA Refnum out"=w490:refnum<visa-resource-name>)  [unwired: 6 in, 1 out]
                n426 = Bundle(cluster=w501, enum16{"Init", "Read", "Stop", "12sec"}."Read", "Data"=w492) -> (w500:T3)
                n427 = Enqueue Element(queue=w502, element=w500, error in (no error)=w499) -> (queue out=w498:refnum<queue>, error out=w497:errorcluster)  [unwired: 1 in, 1 out]
                n428 = Unbundle By Name(w497) -> ("status"=w494:bool)
                n429 = Unbundle By Name(w491) -> ("status"=w493:bool)
                n430 = Compound Arithmetic op=OR ("Opérateur arithmétique")(w493, w494, FALSE) -> (w496:bool)
              }
              event "12sec IR": Value Change {
                n431 = event-data() -> ()  [unwired: 1 in, 6 out]
                n432 = call "Read Continuous Value (SubVI).vi"("error in"=w503, "VISA Refnum in"=w509) -> ("error out"=w507:errorcluster, "nombre"=w508:dbl, "VISA Refnum out"=w506:refnum<visa-resource-name>)  [unwired: 6 in, 1 out]
                n433 = Bundle(cluster=w518, enum16{"Init", "Read", "Stop", "12sec"}."12sec", "Data"=w508) -> (w517:T3)
                n434 = Enqueue Element(queue=w519, element=w517, error in (no error)=w516) -> (queue out=w515:refnum<queue>, error out=w514:errorcluster)  [unwired: 1 in, 1 out]
                n435 = Unbundle By Name(w514) -> ("status"=w511:bool)
                n436 = property on="12sec IR" class="Bool (strict)"("Value"=FALSE ("12sec IR")) -> ()  [unwired: 2 in, 2 out]
                n437 = Unbundle By Name(w507) -> ("status"=w510:bool)
                n438 = Compound Arithmetic op=OR ("Opérateur arithmétique")(w510, w511, FALSE) -> (w513:bool)
              }
              event "stop IR": Value Change {
                n439 = event-data() -> ()  [unwired: 1 in, 6 out]
                n440 = Bundle(cluster=w534, enum16{"Init", "Read", "Stop", "12sec"}."Stop") -> (w530:T3)  [unwired: 1 in]
                n441 = Enqueue Element(queue=w531, element=w530, error in (no error)=w532) -> (queue out=w533:refnum<queue>, error out=w529:errorcluster)  [unwired: 1 in, 1 out]
                n442 = call "Stop Continuous Value (SubVI).vi"("entrée d'erreur"=w523, "Refnum VISA en entrée"=w524) -> ("sortie d'erreur"=w522:errorcluster, "Refnum VISA en sortie"=w521:refnum<visa-resource-name>)
                n443 = Unbundle By Name(w529) -> ("status"=w526:bool)
                n444 = Unbundle By Name(w522) -> ("status"=w525:bool)
                n445 = Compound Arithmetic op=OR ("Opérateur arithmétique")(w525, w526, TRUE) -> (w528:bool)
              }
            }
          }
          n446 = while {
            shift-right: [w539] -> w301
            shift-left: w312 -> [w546]
            shift-right: [w538] -> w302
            shift-left: w300 -> [w540]
            shift-right: [w535] -> _
            shift-left: _ -> [w536]
            stop <- w537 stop-if-true
            n447 = Dequeue Element(queue=w540, error in (no error)=w546) -> (queue out=w541:refnum<queue>, element=w545:T3, error out=w542:errorcluster)  [unwired: 1 in, 1 out]
            n448 = Unbundle(w545) -> (w544:enum16{"Init", "Read", "Stop", "12sec"}, "Data"=w543:dbl)
            n449 = case shown="\"Read\"" w544 {
              tunnel: w536 -> [_ w553 w564 w576]
              tunnel: w543 -> [_ w552 w565 _]
              tunnel: w542 -> [w550 w557 w570 w581]
              tunnel: w541 -> [w548 w555 w568 w580]
              tunnel: [w550 w557 w570 w579] -> w539
              tunnel: [FALSE FALSE FALSE TRUE] -> w537
              tunnel: [w548 w555 w568 w577] -> w538
              tunnel: [dbl[] [] w551 dbl[] [] w576] -> w535
              frame "Init", Default {
              }
              frame "Read" {
                n450 = for {
                  N: 1 -> [_]
                  tunnel: w553 -> [w562]
                  tunnel: [w561] -> w551 if=w558
                  tunnel: w552 -> [w560]
                  n451 = Equal To 0?(x=w560) -> (x = 0?=w559:bool)
                  n452 = Insert Into Array(array=w562, new element=w560) -> (w561:dbl[])  [unwired: 1 in]
                  n453 = Not(x=w559) -> (.not. x?=w558:bool)
                }
                n454 = property on="Tableau IR" class="Tabl (strict)"("Value"=w551) -> ()  [unwired: 2 in, 2 out]
              }
              frame "12sec" {
                n455 = for {
                  N: 1 -> [_]
                  tunnel: w564 -> [w575]
                  tunnel: [w574] -> w563 if=w571
                  tunnel: w565 -> [w573]
                  n456 = Equal To 0?(x=w573) -> (x = 0?=w572:bool)
                  n457 = Insert Into Array(array=w575, new element=w573) -> (w574:dbl[])  [unwired: 1 in]
                  n458 = Not(x=w572) -> (.not. x?=w571:bool)
                }
                n459 = property on="Tableau IR" class="Tabl (strict)"("Value"=w563) -> ()  [unwired: 2 in, 2 out]
              }
              frame "Stop" {
                n460 = Flush Queue(queue=w580, error in (no error)=w581) -> (queue out=w577:refnum<queue>, error out=w579:errorcluster)  [unwired: 1 out]
              }
            }
          }
          n461 = Release Queue(queue=w302, error in (no error)=w301) -> (error out=w309:errorcluster)  [unwired: 1 in, 2 out]
          n462 = Merge Errors(w311, w310, w309) -> (w294:errorcluster)
          n463 = Merge Errors(w294, w293, w292) -> (w291:errorcluster)
        }
        frame Error {
        }
      }
      "sortie d'erreur" <- w283
    }
    frame #2 {
      n464 = property on="sortie d'erreur" class="Clust (strict)"() -> ("Value"=w826:errorcluster)  [unwired: 2 in, 2 out]
      n465 = case shown="Pas d'erreur" w826 {
        selector: w826 -> [_ w918]
        frame No Error {
          n466 = stacked-sequence {
            frame #0 {
              n467 = property on="Start acquisition" class="Bool (strict)"("Visible"=FALSE) -> ()  [unwired: 2 in, 2 out]
              n468 = property on="stop" class="Bool (strict)"("Visible"=FALSE) -> ()  [unwired: 2 in, 2 out]
              n469 = property on="COM Port table" class="Tabl (strict)"() -> ("Value"=w828:refnum<visa-resource-name>[])  [unwired: 2 in, 2 out]
              n470 = property on="Commande onglets" class="Onglet (strict)"("DisabledEnum"=T2."Disabled and Grayed Out" ("Désactivé")) -> ()  [unwired: 2 in, 2 out]
              n471 = for {
                tunnel: w828 -> [w832] mode=indexing
                n472 = call "Port Close (SubVI).vi"("VISA Refnum in"=w832) -> ()  [unwired: 1 in, 2 out]
                n473 = Wait (ms)(milliseconds to wait=u32 500 ("attente (ms)")) -> ()  [unwired: 1 out]
              }
              n474 = property on="Update" class="Ch"("Value"="Closing COM Port" ("Étiquette.Texte")) -> ()  [unwired: 2 in, 2 out]
            }
            frame #1 {
              w834 = enum16{"start", "end", "current"}."end" ("à partir de (0 : start)")
              w835 = i64 0 ("offset (en octets) (0)")
              n475 = property on="Energie UV file (1sec)" class="Ref (strict)"() -> ("Value"=w861:refnum<file>)  [unwired: 2 in, 2 out]
              n476 = property on="Energie UV file (stats)" class="Ref (strict)"() -> ("Value"=w862:refnum<file>)  [unwired: 2 in, 2 out]
              n477 = property on="Puissance depolar file (1sec)" class="Ref (strict)"() -> ("Value"=w863:refnum<file>)  [unwired: 2 in, 2 out]
              n478 = property on="Puissance depolar file (stats)" class="Ref (strict)"() -> ("Value"=w864:refnum<file>)  [unwired: 2 in, 2 out]
              n479 = property on="Energie IR file (1sec)" class="Ref (strict)"() -> ("Value"=w865:refnum<file>)  [unwired: 2 in, 2 out]
              n480 = property on="Energie IR file (stats)" class="Ref (strict)"() -> ("Value"=w866:refnum<file>)  [unwired: 2 in, 2 out]
              n481 = property on="Energy UV file (500pts)" class="Ref (strict)"() -> ("Value"=w838:refnum<file>)  [unwired: 2 in, 2 out]
              n482 = property on="Puissance depolar file (500pts)" class="Ref (strict)"() -> ("Value"=w837:refnum<file>)  [unwired: 2 in, 2 out]
              n483 = property on="Energie IR file (500pts)" class="Ref (strict)"() -> ("Value"=w836:refnum<file>)  [unwired: 2 in, 2 out]
              n484 = Get Date/Time In Seconds() -> (seconds since 1Jan1904=w848:timestamp)
              n485 = Format Date/Time String(time format string (%c)="%d-%m-%Y-%H:%M:%S%3u", seconds (now)=w848) -> (date/time string=w846:string)  [unwired: 1 in]
              n486 = Set File Position(offset (in bytes) (0)=w835, refnum=w861, from (0:start)=w834) -> (refnum out=w854:refnum<file>)  [unwired: 1 in, 1 out]
              n487 = Set File Position(offset (in bytes) (0)=w835, refnum=w862, from (0:start)=w834) -> (refnum out=w853:refnum<file>)  [unwired: 1 in, 1 out]
              n488 = Set File Position(offset (in bytes) (0)=w835, refnum=w863, from (0:start)=w834) -> (refnum out=w852:refnum<file>)  [unwired: 1 in, 1 out]
              n489 = Set File Position(offset (in bytes) (0)=w835, refnum=w864, from (0:start)=w834) -> (refnum out=w851:refnum<file>)  [unwired: 1 in, 1 out]
              n490 = Set File Position(offset (in bytes) (0)=w835, refnum=w865, from (0:start)=w834) -> (refnum out=w850:refnum<file>)  [unwired: 1 in, 1 out]
              n491 = Set File Position(offset (in bytes) (0)=w835, refnum=w866, from (0:start)=w834) -> (refnum out=w849:refnum<file>)  [unwired: 1 in, 1 out]
              n492 = Set File Position(offset (in bytes) (0)=w835, refnum=w838, from (0:start)=w834) -> (refnum out=w843:refnum<file>)  [unwired: 1 in, 1 out]
              n493 = Set File Position(offset (in bytes) (0)=w835, refnum=w837, from (0:start)=w834) -> (refnum out=w844:refnum<file>)  [unwired: 1 in, 1 out]
              n494 = Set File Position(offset (in bytes) (0)=w835, refnum=w836, from (0:start)=w834) -> (refnum out=w845:refnum<file>)  [unwired: 1 in, 1 out]
              n495 = Concatenate Strings(w846) -> (w839:string)
              n496 = Write to Text File(file (use dialog)=w854, text=w839) -> (refnum out=w860:refnum<file>)  [unwired: 2 in, 2 out]
              n497 = Write to Text File(file (use dialog)=w853, text=w839) -> (refnum out=w859:refnum<file>)  [unwired: 2 in, 2 out]
              n498 = Write to Text File(file (use dialog)=w852, text=w839) -> (refnum out=w858:refnum<file>)  [unwired: 2 in, 2 out]
              n499 = Write to Text File(file (use dialog)=w851, text=w839) -> (refnum out=w857:refnum<file>)  [unwired: 2 in, 2 out]
              n500 = Write to Text File(file (use dialog)=w850, text=w839) -> (refnum out=w856:refnum<file>)  [unwired: 2 in, 2 out]
              n501 = Write to Text File(file (use dialog)=w849, text=w839) -> (refnum out=w855:refnum<file>)  [unwired: 2 in, 2 out]
              n502 = Write to Text File(file (use dialog)=w843, text=w839) -> (refnum out=w840:refnum<file>)  [unwired: 2 in, 2 out]
              n503 = Write to Text File(file (use dialog)=w844, text=w839) -> (refnum out=w841:refnum<file>)  [unwired: 2 in, 2 out]
              n504 = Write to Text File(file (use dialog)=w845, text=w839) -> (refnum out=w842:refnum<file>)  [unwired: 2 in, 2 out]
              n505 = Close File(refnum=w860) -> ()  [unwired: 1 in, 2 out]
              n506 = Close File(refnum=w859) -> ()  [unwired: 1 in, 2 out]
              n507 = Close File(refnum=w858) -> ()  [unwired: 1 in, 2 out]
              n508 = Close File(refnum=w857) -> ()  [unwired: 1 in, 2 out]
              n509 = Close File(refnum=w856) -> ()  [unwired: 1 in, 2 out]
              n510 = Close File(refnum=w855) -> ()  [unwired: 1 in, 2 out]
              n511 = Close File(refnum=w840) -> ()  [unwired: 1 in, 2 out]
              n512 = Close File(refnum=w841) -> ()  [unwired: 1 in, 2 out]
              n513 = Close File(refnum=w842) -> ()  [unwired: 1 in, 2 out]
            }
            frame #2 {
              n514 = stacked-sequence {
                tunnel: [w885 _ _] -> w867
                tunnel: [_ w888 _] -> w868
                tunnel: [_ _ w903] -> w869
                frame #0 {
                  n515 = property on="Auto Scale (Energie UV)" class="Bool (strict)"() -> ("Value"=w877:bool)  [unwired: 2 in, 2 out]
                  n516 = property on="Multiplier (Energie UV)" class="NumNb (strict)"() -> ("Value"=w879:sgl)  [unwired: 2 in, 2 out]
                  n517 = property on="Trigger Level (% of Scale) (Energie UV)" class="NumNb (strict)"() -> ("Value"=w878:dbl)  [unwired: 2 in, 2 out]
                  n518 = property on="COM port (Energie UV)" class="NumNb (strict)"() -> ("Value"=w884:i64)  [unwired: 2 in, 2 out]
                  n519 = property on="Wavelength (nm) (Energie UV)" class="NumNb (strict)"() -> ("Value"=w883:u32)  [unwired: 2 in, 2 out]
                  n520 = property on="Offset (Energie UV)" class="NumNb (strict)"() -> ("Value"=w882:sgl)  [unwired: 2 in, 2 out]
                  n521 = property on="Scale (Watt or Joule) (Energie UV)" class="MDér (strict)"() -> ("Value"=w874:i32)  [unwired: 2 in, 2 out]
                  n522 = Boolean To (0,1)(Boolean=w877) -> (0, 1=w876:i16)
                  n523 = To Double Precision Float(number=w879) -> (double precision float=w871:dbl)
                  n524 = To Double Precision Float(number=w882) -> (double precision float=w872:dbl)
                  n525 = To Double Precision Float(number=w876) -> (double precision float=w875:dbl)
                  n526 = To Double Precision Float(number=w874) -> (double precision float=w873:dbl)
                  n527 = To Double Precision Float(number=w884) -> (double precision float=w881:dbl)
                  n528 = To Double Precision Float(number=w883) -> (double precision float=w880:dbl)
                  n529 = Build Array(w881, w880, w872, w871, w878, w875, w873) -> (w885:dbl[])
                }
                frame #1 {
                  n530 = property on="Auto Scale (Puissance depolar)" class="Bool (strict)"() -> ("Value"=w893:bool)  [unwired: 2 in, 2 out]
                  n531 = property on="Multiplier (Puissance depolar)" class="NumNb (strict)"() -> ("Value"=w895:sgl)  [unwired: 2 in, 2 out]
                  n532 = property on="Trigger Level (% of Scale) (Puissance depolar)" class="NumNb (strict)"() -> ("Value"=w894:dbl)  [unwired: 2 in, 2 out]
                  n533 = property on="COM Port (Puissance depolar)" class="NumNb (strict)"() -> ("Value"=w900:i64)  [unwired: 2 in, 2 out]
                  n534 = property on="Wavelength (nm) (Puissance depolar)" class="NumNb (strict)"() -> ("Value"=w899:u32)  [unwired: 2 in, 2 out]
                  n535 = property on="Offset (Puissance depolar)" class="NumNb (strict)"() -> ("Value"=w898:sgl)  [unwired: 2 in, 2 out]
                  n536 = property on="Scale (Watt or Joule) (Puissance depolar)" class="MDér (strict)"() -> ("Value"=w890:u16)  [unwired: 2 in, 2 out]
                  n537 = Boolean To (0,1)(Boolean=w893) -> (0, 1=w892:i16)
                  n538 = To Double Precision Float(number=w898) -> (double precision float=w887:dbl)
                  n539 = To Double Precision Float(number=w895) -> (double precision float=w886:dbl)
                  n540 = To Double Precision Float(number=w892) -> (double precision float=w891:dbl)
                  n541 = To Double Precision Float(number=w890) -> (double precision float=w889:dbl)
                  n542 = To Double Precision Float(number=w900) -> (double precision float=w897:dbl)
                  n543 = To Double Precision Float(number=w899) -> (double precision float=w896:dbl)
                  n544 = Build Array(w897, w896, w887, w886, w894, w891, w889) -> (w888:dbl[])
                }
                frame #2 {
                  n545 = property on="Auto Scale (Energie IR)" class="Bool (strict)"() -> ("Value"=w908:bool)  [unwired: 2 in, 2 out]
                  n546 = property on="Multiplier (Energie IR)" class="NumNb (strict)"() -> ("Value"=w910:sgl)  [unwired: 2 in, 2 out]
                  n547 = property on="Trigger Level (% of Scale) (Energie IR)" class="NumNb (strict)"() -> ("Value"=w909:dbl)  [unwired: 2 in, 2 out]
                  n548 = property on="COM Port (Energie IR)" class="NumNb (strict)"() -> ("Value"=w915:i64)  [unwired: 2 in, 2 out]
                  n549 = property on="Wavelength (nm) (Energie IR)" class="NumNb (strict)"() -> ("Value"=w914:u32)  [unwired: 2 in, 2 out]
                  n550 = property on="Offset (Energie IR)" class="NumNb (strict)"() -> ("Value"=w913:sgl)  [unwired: 2 in, 2 out]
                  n551 = property on="Scale (Watt or Joule) (Energie IR)" class="MDér (strict)"() -> ("Value"=w905:u16)  [unwired: 2 in, 2 out]
                  n552 = Boolean To (0,1)(Boolean=w908) -> (0, 1=w907:i16)
                  n553 = To Double Precision Float(number=w910) -> (double precision float=w901:dbl)
                  n554 = To Double Precision Float(number=w913) -> (double precision float=w902:dbl)
                  n555 = To Double Precision Float(number=w907) -> (double precision float=w906:dbl)
                  n556 = To Double Precision Float(number=w905) -> (double precision float=w904:dbl)
                  n557 = To Double Precision Float(number=w915) -> (double precision float=w912:dbl)
                  n558 = To Double Precision Float(number=w914) -> (double precision float=w911:dbl)
                  n559 = Build Array(w912, w911, w902, w901, w909, w906, w904) -> (w903:dbl[])
                }
              }
              n560 = property on="file path" class="Chm"() -> ("Value"=w870:path)  [unwired: 2 in, 2 out]
              n561 = call "Write User File (SubVI).vi"("configuration file path"=w870, "User file contents Energie UV"=w867, "User file contents Puissance depolar"=w868, "User file contents Energie IR"=w869) -> ()  [unwired: 22 in, 2 out]
            }
            frame #3 {
              n562 = flat-sequence {
                frame #0 {
                  n563 = property on="Update" class="Ch"("Value"="End" ("Étiquette.Texte")) -> ()  [unwired: 2 in, 2 out]
                }
                frame #1 {
                  n564 = Stop(stop? (T)=TRUE ("flag")) -> ()
                }
              }
            }
          }
        }
        frame Error {
          n565 = stacked-sequence {
            tunnel: w918 -> [_ w922]
            frame #0 {
              n566 = property on="Start acquisition" class="Bool (strict)"("Visible"=TRUE) -> ()  [unwired: 2 in, 2 out]
              n567 = property on="stop" class="Bool (strict)"("Visible"=FALSE) -> ()  [unwired: 2 in, 2 out]
              n568 = property on="Commande onglets" class="Onglet (strict)"("DisabledEnum"=T2."Enabled" ("Désactivé")) -> ()  [unwired: 2 in, 2 out]
            }
            frame #1 {
              n569 = flat-sequence {
                tunnel: w922 -> [w923]
                frame #0 {
                  n570 = call <vilib>:"General Error Handler.vi"("error in (no error)"=w923) -> ()  [unwired: 10 in, 5 out]
                }
                frame #1 {
                  w924 = TRUE ("stop ? (V)")
                  n571 = Stop(stop? (T)=w924) -> ()
                  n572 = Request Deallocation(w924) -> ()
                }
              }
            }
          }
        }
      }
    }
  }
